vi "main 9th.vi"() -> ()   [LabVIEW 2015]
uses:
  Abort.vi
panel:
  out "number of function calls":i32
  out "External Trigger":bool
  out "x-y":u32
  in  "Live Image Display 2":refnum<k7>(container)
  in  "Live Image Display":refnum<k7>(container)
  in  "Initial guess values 2":dbl[](array[numeric])
  in  "Fitting Results Save Path 2":string[](array[string])
  out "Current File Num":u16
  out "Two Cameras ?":bool
  out "3":u32
  out "2":u32
  out "5":u32
  out "4":u32
  out "From OD fit?":bool
  in  "Fitting Results Save Path":string[](array[string])
  in  "Initial guess values":dbl[](array[numeric])
  out "Latest image data":dbl[][](array[numeric])
  in  "Fitting Type":u16(ring)
  in  "Force Guess?":bool
  in  "Abort":bool
  in  "FFT Auto?":bool[](array[boolean]) caption="Auto?"
  in  "Ring":u16(ring) items=["Atom", "Light", "Dark", "OD"]
  in  "Select Cam Fit":bool[](array[boolean])
  in  "Binning Average?":bool caption="Average?"
  in  "FFT Process":bool caption="Process"
  in  "Threshold":dbl
  out "Label":string[](array[string])
  in  "Pics to show in IJ":bool[][](array[boolean])
  out "Trigger":bool
  in  "Save Fit":bool
  out "best fit parameters 2":dbl[][](array[numeric])
  in  "Binning Enabled":bool
  in  "Binning":u8[](array[numeric])
  out "ROI Width":u16[](array[numeric])
  out "ROI Height":u16[](array[numeric])
  out "best fit parameters":dbl[][](array[numeric])
  in  "Reset Cam Buffer":bool
  out "OD image":u16[][](graph)
  out "XY图":cluster{i32[], dbl[]}[](graph)
  in  "OD fit":bool caption="Open"
  in  "OD Num":i32
  out "Fitting...":bool
  in  "Exit":bool
  out "XY图 2":cluster{i32[], dbl[]}[](graph)
  in  "Fit":bool
  in  "Open File":bool
  in  "Auto Fit":bool
  in  "Stop":bool
  in  "Aquire":bool
  in  "Fitting Config":bool
  in  "Camera Config":bool
  in  "Initialize":bool
  # "Cam1"
  # "Cam2"
  # "Atom"
  # "Light"
  # "Dark"
  # "OD"
  # "FFT and Low Pass"
  # "Na"
  # "Rb"
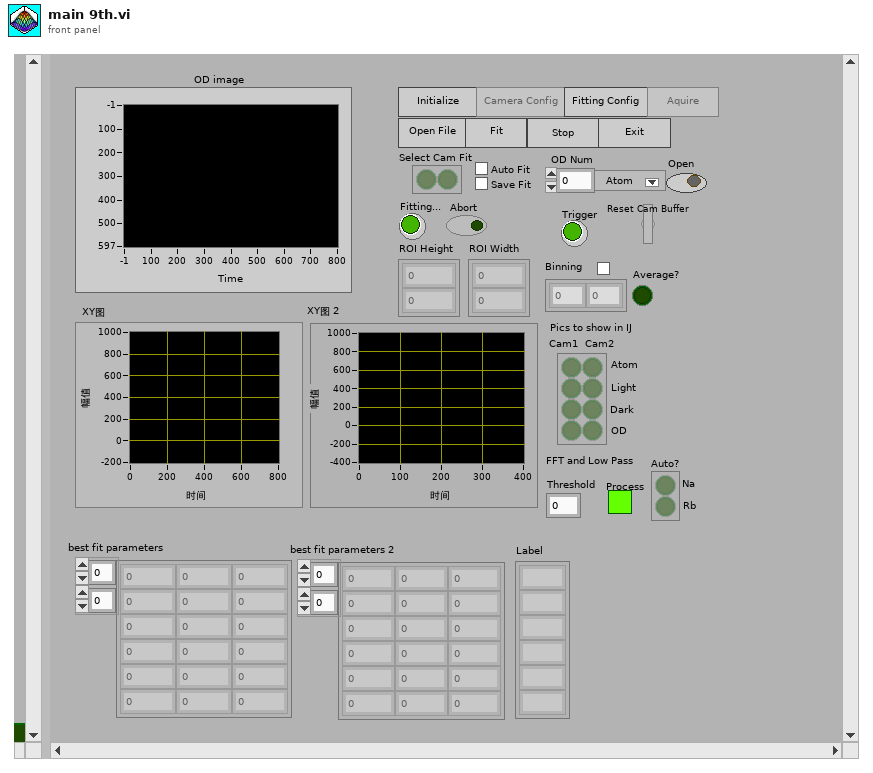
[diagram p1: front panel]
types:
  T1 = enum8{"Enabled", "Disabled", "Disabled and Grayed Out"}
  T2 = enum16{"Left Button", "Center Button", "Right Button", "Window Close"}
  T3 = typedef "Image Type" = u32
  T4 = typedef "IMAQ Image.ctl" = refnum<image>
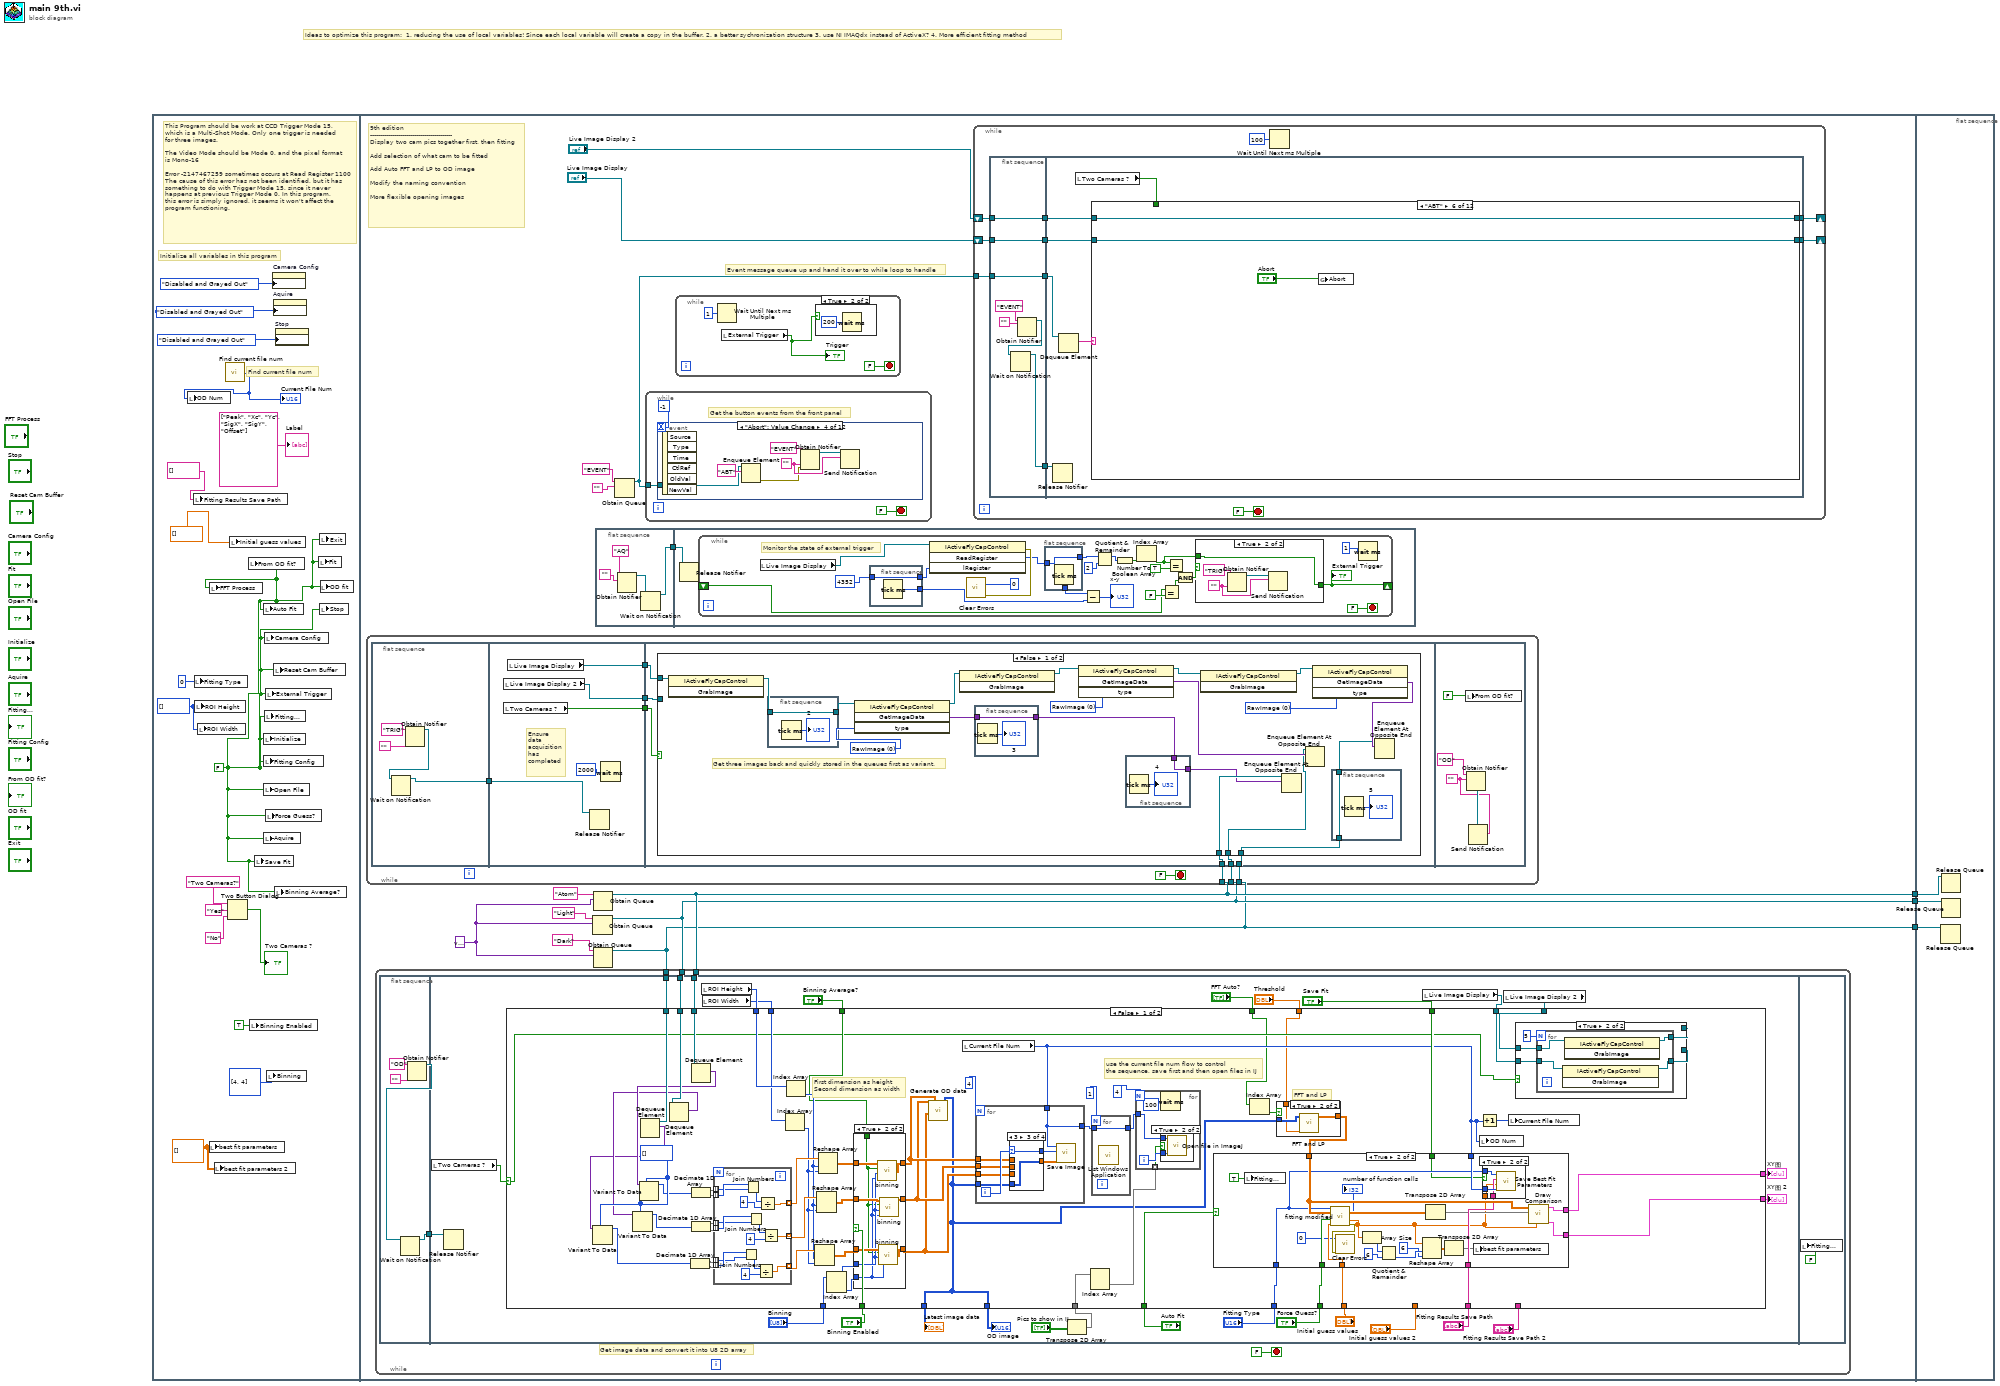
[diagram p0: block diagram]
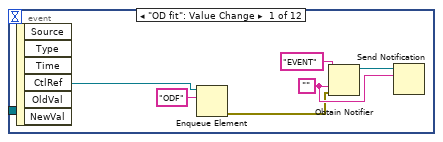
[diagram p3: hidden frame]
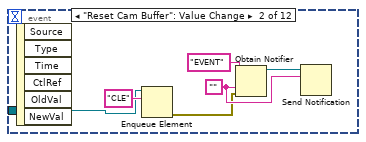
[diagram p4: hidden frame]
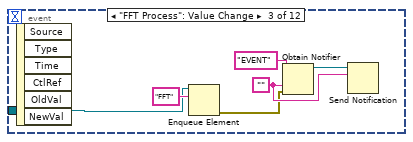
[diagram p5: hidden frame]
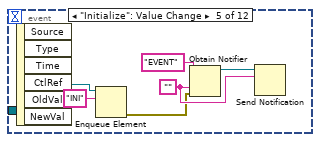
[diagram p6: hidden frame]
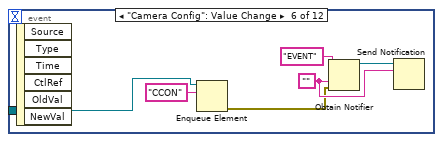
[diagram p7: hidden frame]
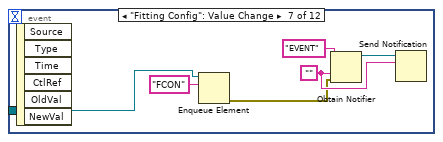
[diagram p8: hidden frame]
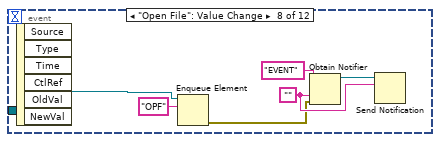
[diagram p9: hidden frame]
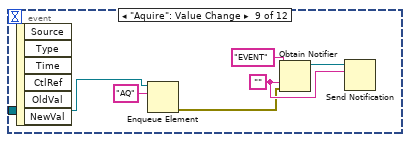
[diagram p10: hidden frame]
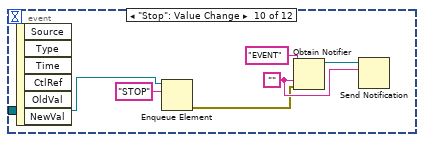
[diagram p11: hidden frame]
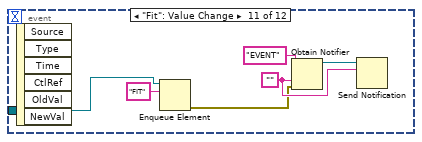
[diagram p12: hidden frame]
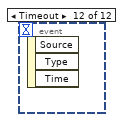
[diagram p13: hidden frame]
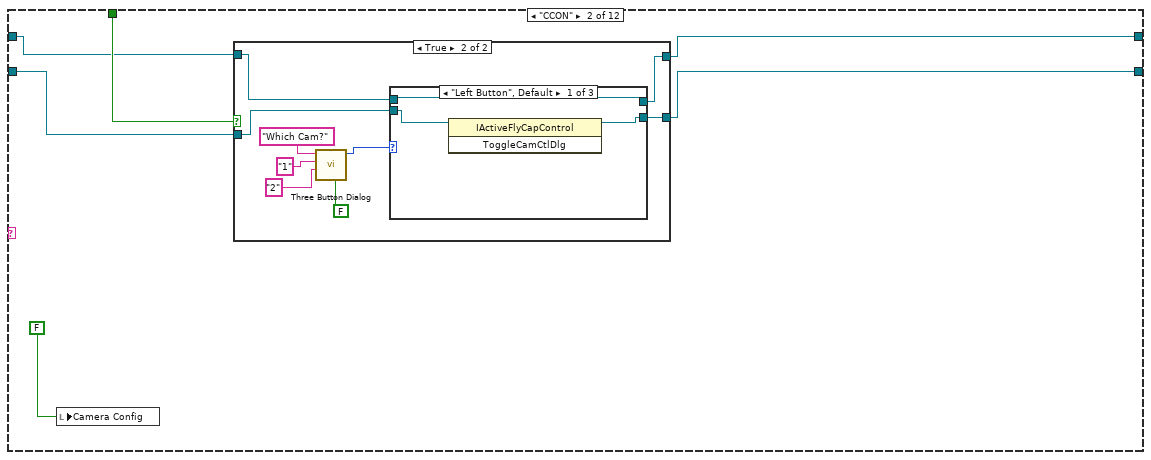
[diagram p15: hidden frame]
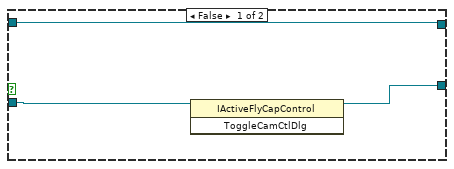
[diagram p16: hidden frame]
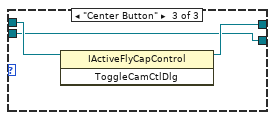
[diagram p18: hidden frame]
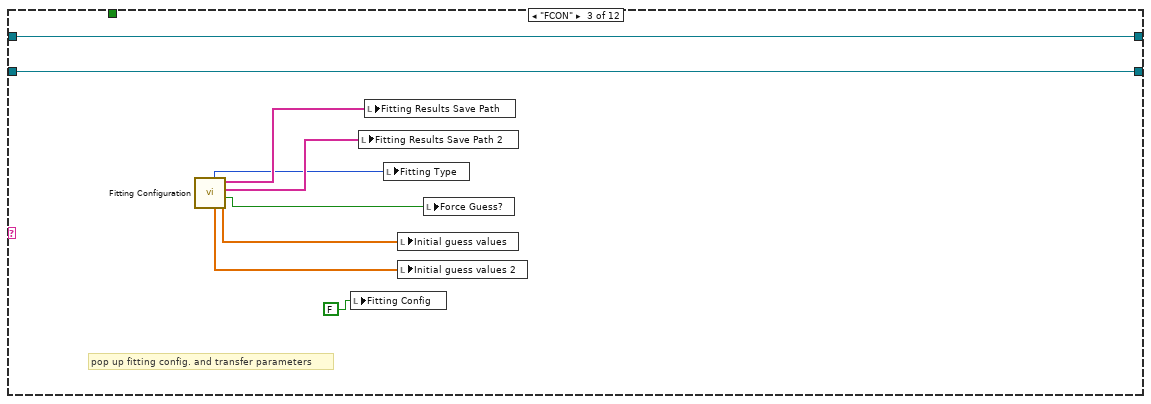
[diagram p19: hidden frame]
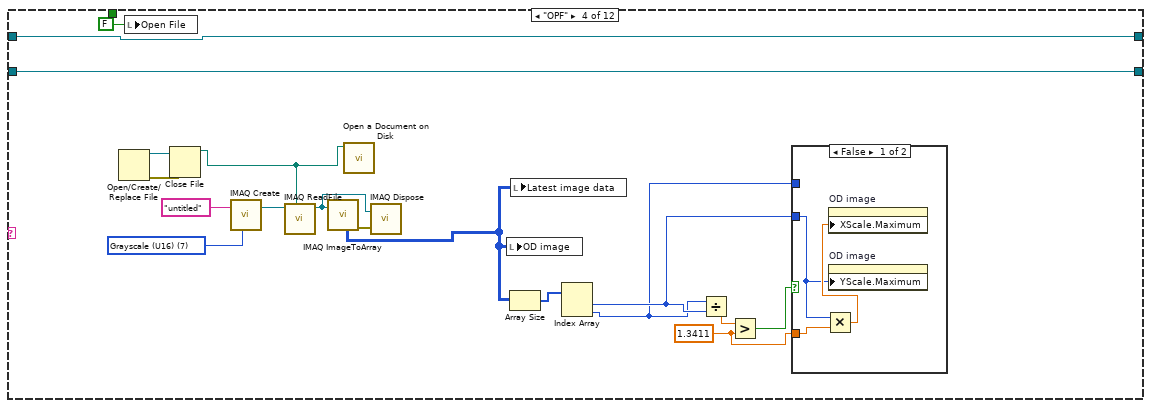
[diagram p20: hidden frame]
diagram:
  # "Ideas to optimize this program:  1. reducing the use of local variables! Since each local variable will create a copy in the buffer. 2. a better sychronization structure 3. use NI IMAQdx instead of ActiveX? 4. More efficient fitting method"
  n1 = flat-sequence {
    tunnel: [w29] -> w3
    tunnel: [w28] -> w2
    tunnel: [w27] -> w1
    tunnel: w3 -> [w1041]
    tunnel: w2 -> [w1040]
    tunnel: w1 -> [w1039]
    frame #0 {
      w6 = dbl[][] [] ("best fit parameters")
      w10 = u16[] [] ("ROI Height")
      w5 = FALSE ("Aquire")
      # "This Program should be work at CCD Trigger Mode 15,\nwhich is a Multi-Shot Mode. Only one trigger is needed\nfor three images. \n\nThe Video Mode should be Mode 0, and the pixel format\nis Mono-16\n\nError -2147467259 sometimes occurs at Read Register 1100\nThe cause of this error has not been identified, but it has\nsomething to do with Trigger Mode 15, since it never \nhappens at previous Trigger Mode 0. In this program,\nthis error is simply ignored, it seems it won't affect the \nprogram functioning."
      # "Find current file num"
      # "Initialize all variables in this program"
      n2 = local write "Fitting Results Save Path"(string[] [] ("Fitting Results Save Path")) -> ()
      n3 = local write "Fitting Type"(0 ("OD num")) -> ()
      n4 = local write "ROI Height"(w10) -> ()
      n5 = local write "ROI Width"(w10) -> ()
      n6 = local write "best fit parameters"(w6) -> ()
      n7 = local write "FFT Process"(w5) -> ()
      n8 = local write "best fit parameters 2"(w6) -> ()
      n9 = call "Find current file num.vi"() -> ("Current File Num"=w4:u16)  [unwired: 2 in]
      "Current File Num" <- w4
      n10 = local write "OD Num"(w4) -> ()
      n11 = Two Button Dialog(message="Two Cameras?" ("消息"), 1:"No" ("F按钮名称（“取消”）"), 2:"Yes" ("T按钮名称（“确定”）")) -> (T button?=→"Two Cameras ?":bool)
      n12 = local write "Initial guess values"(dbl[] [] ("Best fit parameters")) -> ()
      n13 = local write "From OD fit?"(w5) -> ()
      n14 = local write "Binning Enabled"(TRUE ("Binning Enabled")) -> ()
      n15 = local write "Save Fit"(w5) -> ()
      n16 = local write "Auto Fit"(w5) -> ()
      n17 = local write "Initialize"(w5) -> ()
      n18 = local write "Fitting Config"(w5) -> ()
      n19 = local write "Open File"(w5) -> ()
      n20 = local write "Aquire"(w5) -> ()
      n21 = local write "Camera Config"(w5) -> ()
      n22 = local write "Fitting..."(w5) -> ()
      n23 = local write "Force Guess?"(w5) -> ()
      n24 = local write "External Trigger"(w5) -> ()
      n25 = local write "Binning"(u8[] [4, 4] ("Binning")) -> ()
      n26 = property on="Camera Config" class="Bool (strict)"("DisabledEnum"=T1."Disabled and Grayed Out" ("禁用")) -> ()  [unwired: 2 in, 2 out]
      n27 = property on="Aquire" class="Bool (strict)"("DisabledEnum"=T1."Disabled and Grayed Out" ("禁用")) -> ()  [unwired: 2 in, 2 out]
      n28 = local write "Reset Cam Buffer"(w5) -> ()
      n29 = local write "Binning Average?"(w5) -> ()
      n30 = property on="Stop" class="Bool (strict)"("DisabledEnum"=T1."Disabled and Grayed Out" ("禁用")) -> ()  [unwired: 2 in, 2 out]
      n31 = local write "Fit"(w5) -> ()
      n32 = local write "Exit"(w5) -> ()
      n33 = local write "Stop"(w5) -> ()
      n34 = local write "OD fit"(w5) -> ()
      "Label" <- string[] ["Peak", "Xc", "Yc", "SigX", "SigY", "Offset"] ("Label")
    }
    frame #1 {
      w23 = variant
      # "9th edition\n-----------------------------------------\nDisplay two cam pics together first, then fitting\n\nAdd selection of what cam to be fitted\n\nAdd Auto FFT and LP to OD image\n\nModify the naming convention\n\nMore flexible opening images"
      # "Event message queue up and hand it over to while loop to handle"
      n35 = Obtain Queue(name (unnamed)="Light" ("名称（未命名）"), element data type=w23) -> (queue out=w28:refnum<queue>)  [unwired: 3 in, 2 out]
      n36 = Obtain Queue(name (unnamed)="Atom" ("名称（未命名）"), element data type=w23) -> (queue out=w29:refnum<queue>)  [unwired: 3 in, 2 out]
      n37 = Obtain Queue(name (unnamed)="Dark" ("名称（未命名）"), element data type=w23) -> (queue out=w27:refnum<queue>)  [unwired: 3 in, 2 out]
      n38 = while {
        tunnel: w29 -> [w949]
        tunnel: w28 -> [w948]
        tunnel: w27 -> [w947]
        stop <- FALSE stop-if-true
        n39 = flat-sequence {
          tunnel: [w951] -> w950
          tunnel: w950 -> [w959]
          tunnel: [w958] -> w945
          tunnel: [w957] -> w944
          tunnel: [w956] -> w943
          tunnel: w949 -> [w965]
          tunnel: w948 -> [w964]
          tunnel: w947 -> [w963]
          tunnel: w945 -> [w962]
          tunnel: w944 -> [w961]
          tunnel: w943 -> [w960]
          frame #0 {
            n40 = Obtain Notifier(name (unnamed)="TRIG" ("名称（未命名）"), notification data type="") -> (notifier out=w952:refnum<notifier>)  [unwired: 2 in, 2 out]
            n41 = Wait on Notification(notifier=w952) -> (notifier out=w951:refnum<notifier>)  [unwired: 3 in, 3 out]
          }
          frame #1 {
            # "Ensure\ndata\nacquisition\nhas \ncompleted"
            n42 = local read "Live Image Display 2"() -> (w957:refnum<k7>)
            n43 = local read "Two Cameras ?"() -> (w956:bool)
            n44 = local read "Live Image Display"() -> (w958:refnum<k7>)
            n45 = Release Notifier(notifier=w959) -> ()  [unwired: 2 in, 3 out]
            n46 = Wait (ms)(milliseconds to wait=u32 2000) -> ()  [unwired: 1 out]
          }
          frame #2 {
            n47 = case shown="False" w960 {
              tunnel: w965 -> [w983 w998]
              tunnel: w964 -> [w974 w997]
              tunnel: w963 -> [w971 w996]
              tunnel: w962 -> [w967 w994]
              tunnel: w961 -> [_ w993]
              frame False {
                w969 = 0 items=["RawImage", "ColorProcessedImage"] ("type")
                w970 = 0 items=["RawImage", "ColorProcessedImage"] ("type")
                w984 = 0 items=["RawImage", "ColorProcessedImage"] ("type")
                # "Get three images back and quickly stored in the queues first as variant."
                n48 = invoke class="IActiveFlyCapControl" method="GrabImage"(reference=w967) -> (reference out=w966:refnum<k7>)  [unwired: 2 in, 2 out]
                n49 = flat-sequence {
                  tunnel: w966 -> [w987]
                  tunnel: [w987] -> w981
                  frame #0 {
                    n50 = Tick Count (ms)() -> (millisecond timer value=→"2":u32)
                  }
                }
                n51 = invoke class="IActiveFlyCapControl" method="GetImageData"(reference=w981, "type"=w984) -> (reference out=w978:refnum<k7>, "GetImageData"=w980:variant)  [unwired: 2 in, 2 out]
                n52 = invoke class="IActiveFlyCapControl" method="GrabImage"(reference=w978) -> (reference out=w977:refnum<k7>)  [unwired: 2 in, 2 out]
                n53 = flat-sequence {
                  tunnel: [w985] -> w979
                  tunnel: w980 -> [w985]
                  frame #0 {
                    n54 = Tick Count (ms)() -> (millisecond timer value=→"3":u32)
                  }
                }
                n55 = invoke class="IActiveFlyCapControl" method="GetImageData"(reference=w977, "type"=w970) -> (reference out=w976:refnum<k7>, "GetImageData"=w975:variant)  [unwired: 2 in, 2 out]
                n56 = flat-sequence {
                  tunnel: w979 -> [w992]
                  tunnel: [w992] -> w982
                  frame #0 {
                    n57 = Tick Count (ms)() -> (millisecond timer value=→"4":u32)
                  }
                }
                n58 = invoke class="IActiveFlyCapControl" method="GrabImage"(reference=w976) -> (reference out=w973:refnum<k7>)  [unwired: 2 in, 2 out]
                n59 = Enqueue Element At Opposite End(queue=w983, element=w982) -> ()  [unwired: 2 in, 3 out]
                n60 = Enqueue Element At Opposite End(queue=w974, element=w975) -> ()  [unwired: 2 in, 3 out]
                n61 = invoke class="IActiveFlyCapControl" method="GetImageData"(reference=w973, "type"=w969) -> ("GetImageData"=w972:variant)  [unwired: 2 in, 3 out]
                n62 = flat-sequence {
                  tunnel: w971 -> [w989]
                  tunnel: [w989] -> w968
                  frame #0 {
                    n63 = Tick Count (ms)() -> (millisecond timer value=→"5":u32)
                  }
                }
                n64 = Enqueue Element At Opposite End(queue=w968, element=w972) -> ()  [unwired: 2 in, 3 out]
              }
              frame True {
                # "Since element is added at the front of the queue, queue cam2 first then cam1"
                n65 = for {
                  N: 2 -> [_]
                  tunnel: w998 -> [w1004]
                  tunnel: w997 -> [w1003]
                  tunnel: w996 -> [w1002]
                  tunnel: w994 -> [w1000]
                  tunnel: w993 -> [w999]
                  i -> [w1001]
                  n66 = case shown="0, Default" w1001 {
                    tunnel: w1004 -> [w1008 w1024]
                    tunnel: w1003 -> [w1007 w1023]
                    tunnel: w1002 -> [w1006 w1022]
                    tunnel: w1000 -> [_ w1021]
                    tunnel: w999 -> [w1005 _]
                    frame 0, Default {
                      w1011 = 0 items=["RawImage", "ColorProcessedImage"] ("type")
                      w1012 = 0 items=["RawImage", "ColorProcessedImage"] ("type")
                      w1019 = 0 items=["RawImage", "ColorProcessedImage"] ("type")
                      # "Get three images back and quickly stored in the queues first as variant."
                      n67 = invoke class="IActiveFlyCapControl" method="GrabImage"(reference=w1005) -> (reference out=w1010:refnum<k7>)  [unwired: 2 in, 2 out]
                      n68 = invoke class="IActiveFlyCapControl" method="GetImageData"(reference=w1010, "type"=w1019) -> (reference out=w1018:refnum<k7>, "GetImageData"=w1009:variant)  [unwired: 2 in, 2 out]
                      n69 = invoke class="IActiveFlyCapControl" method="GrabImage"(reference=w1018) -> (reference out=w1017:refnum<k7>)  [unwired: 2 in, 2 out]
                      n70 = invoke class="IActiveFlyCapControl" method="GetImageData"(reference=w1017, "type"=w1012) -> (reference out=w1016:refnum<k7>, "GetImageData"=w1015:variant)  [unwired: 2 in, 2 out]
                      n71 = invoke class="IActiveFlyCapControl" method="GrabImage"(reference=w1016) -> (reference out=w1014:refnum<k7>)  [unwired: 2 in, 2 out]
                      n72 = invoke class="IActiveFlyCapControl" method="GetImageData"(reference=w1014, "type"=w1011) -> ("GetImageData"=w1013:variant)  [unwired: 2 in, 3 out]
                      n73 = Enqueue Element At Opposite End(queue=w1008, element=w1009) -> ()  [unwired: 2 in, 3 out]
                      n74 = Enqueue Element At Opposite End(queue=w1007, element=w1015) -> ()  [unwired: 2 in, 3 out]
                      n75 = Enqueue Element At Opposite End(queue=w1006, element=w1013) -> ()  [unwired: 2 in, 3 out]
                    }
                    frame 1 {
                      w1027 = 0 items=["RawImage", "ColorProcessedImage"] ("type")
                      w1028 = 0 items=["RawImage", "ColorProcessedImage"] ("type")
                      w1034 = 0 items=["RawImage", "ColorProcessedImage"] ("type")
                      # "Get three images back and quickly stored in the queues first as variant."
                      n76 = invoke class="IActiveFlyCapControl" method="GrabImage"(reference=w1021) -> (reference out=w1026:refnum<k7>)  [unwired: 2 in, 2 out]
                      n77 = invoke class="IActiveFlyCapControl" method="GetImageData"(reference=w1026, "type"=w1034) -> (reference out=w1033:refnum<k7>, "GetImageData"=w1025:variant)  [unwired: 2 in, 2 out]
                      n78 = invoke class="IActiveFlyCapControl" method="GrabImage"(reference=w1033) -> (reference out=w1032:refnum<k7>)  [unwired: 2 in, 2 out]
                      n79 = invoke class="IActiveFlyCapControl" method="GetImageData"(reference=w1032, "type"=w1028) -> (reference out=w1031:refnum<k7>, "GetImageData"=w1030:variant)  [unwired: 2 in, 2 out]
                      n80 = invoke class="IActiveFlyCapControl" method="GrabImage"(reference=w1031) -> (reference out=w1020:refnum<k7>)  [unwired: 2 in, 2 out]
                      n81 = invoke class="IActiveFlyCapControl" method="GetImageData"(reference=w1020, "type"=w1027) -> ("GetImageData"=w1029:variant)  [unwired: 2 in, 3 out]
                      n82 = Enqueue Element At Opposite End(queue=w1024, element=w1025) -> ()  [unwired: 2 in, 3 out]
                      n83 = Enqueue Element At Opposite End(queue=w1023, element=w1030) -> ()  [unwired: 2 in, 3 out]
                      n84 = Enqueue Element At Opposite End(queue=w1022, element=w1029) -> ()  [unwired: 2 in, 3 out]
                    }
                  }
                }
              }
            }
          }
          frame #3 {
            w1036 = ""
            n85 = local write "From OD fit?"(FALSE ("From OD fit?")) -> ()
            n86 = Obtain Notifier(name (unnamed)="OD" ("名称（未命名）"), notification data type=w1036) -> (notifier out=w1038:refnum<notifier>)  [unwired: 2 in, 2 out]
            n87 = Send Notification(notification=w1036, notifier=w1038) -> ()  [unwired: 1 in, 2 out]
          }
        }
      }
      n88 = while {
        tunnel: w29 -> [w451]
        tunnel: w28 -> [w450]
        tunnel: w27 -> [w449]
        stop <- FALSE stop-if-true
        # "Get image data and convert it into U8 2D array"
        n89 = flat-sequence {
          tunnel: [w453] -> w452
          tunnel: w452 -> [w481]
          tunnel: w451 -> [w484]
          tunnel: w450 -> [w483]
          tunnel: w449 -> [w482]
          frame #0 {
            n90 = Obtain Notifier(name (unnamed)="OD" ("名称（未命名）"), notification data type="") -> (notifier out=w454:refnum<notifier>)  [unwired: 2 in, 2 out]
            n91 = Wait on Notification(notifier=w454) -> (notifier out=w453:refnum<notifier>)  [unwired: 3 in, 3 out]
          }
          frame #1 {
            n92 = local read "Two Cameras ?"() -> (w480:bool)
            n93 = Release Notifier(notifier=w481) -> ()  [unwired: 2 in, 3 out]
            n94 = local read "ROI Height"() -> (w477:u16[])
            n95 = local read "ROI Width"() -> (w476:u16[])
            n96 = Transpose 2D Array(2D array="Pics to show in IJ") -> (transposed array=w463:bool[][])
            n97 = local read "Live Image Display"() -> (w459:refnum<k7>)
            n98 = local read "Live Image Display 2"() -> (w460:refnum<k7>)
            n99 = case shown="False" w480 {
              selector: w480 -> [w490 _]
              tunnel: w484 -> [w542 w682]
              tunnel: w483 -> [w541 w681]
              tunnel: w482 -> [w540 w680]
              tunnel: "Binning" -> [w509 w679]
              tunnel: "Binning Enabled" -> [w508 w678]
              tunnel: w477 -> [w507 w677]
              tunnel: w476 -> [w506 w676]
              tunnel: [w489 w675] -> w475
              tunnel: [w489 w675] -> w474
              tunnel: "Auto Fit" -> [w505 w674]
              tunnel: "Initial guess values" -> [w504 w663]
              tunnel: "Force Guess?" -> [w503 w664]
              tunnel: "Fitting Type" -> [w502 w673]
              tunnel: "Fitting Results Save Path" -> [w501 w660]
              tunnel: [w499 w656] -> w468
              tunnel: [w498 w655] -> w467
              tunnel: "Fitting Results Save Path 2" -> [_ w659]
              tunnel: "Initial guess values 2" -> [_ w658]
              tunnel: "Save Fit" -> [w497 w662]
              tunnel: w463 -> [w496 w671]
              tunnel: "Binning Average?" -> [w494 w670]
              tunnel: w460 -> [w492 w668]
              tunnel: w459 -> [w491 w669]
              tunnel: "Threshold" -> [w485 w647]
              tunnel: "FFT Auto?" -> [w488 w646]
              frame False {
                w525 = u8[] []
                # "FFT and LP"
                # "First dimension as height\nSecond dimension as width"
                # "use the current file num flow to control \nthe sequence, save first and then open files in IJ"
                n100 = Dequeue Element(queue=w540) -> (element=w523:variant)  [unwired: 2 in, 3 out]
                n101 = Variant To Data(type=w525, Variant=w523) -> (data=w520:u8[])  [unwired: 1 in, 1 out]
                n102 = Dequeue Element(queue=w541) -> (element=w524:variant)  [unwired: 2 in, 3 out]
                n103 = Variant To Data(type=w525, Variant=w524) -> (data=w521:u8[])  [unwired: 1 in, 1 out]
                n104 = Decimate 1D Array(w520) -> (w531:u8[], w530:u8[])
                n105 = Dequeue Element(queue=w542) -> (element=w526:variant)  [unwired: 2 in, 3 out]
                n106 = Variant To Data(type=w525, Variant=w526) -> (data=w522:u8[])  [unwired: 1 in, 1 out]
                n107 = Decimate 1D Array(w522) -> (w535:u8[], w534:u8[])
                n108 = Decimate 1D Array(w521) -> (w533:u8[], w532:u8[])
                n109 = for {
                  tunnel: [w589] -> w529 mode=indexing
                  tunnel: w535 -> [w579] mode=indexing
                  tunnel: w534 -> [w580] mode=indexing
                  tunnel: w533 -> [w581] mode=indexing
                  tunnel: w532 -> [w582] mode=indexing
                  tunnel: w531 -> [w583] mode=indexing
                  tunnel: w530 -> [w584] mode=indexing
                  tunnel: [w578] -> w528 mode=indexing
                  tunnel: [w577] -> w527 mode=indexing
                  n110 = Join Numbers(hi=w584, lo=w583) -> ((hi.lo)=w586:u16)
                  n111 = Join Numbers(hi=w580, lo=w579) -> ((hi.lo)=w591:u16)
                  n112 = Join Numbers(hi=w582, lo=w581) -> ((hi.lo)=w588:u16)
                  n113 = Divide(x=w586, y=u16 4) -> (x/y=w577:dbl)
                  n114 = Divide(x=w591, y=u16 4) -> (x/y=w589:dbl)
                  n115 = Divide(x=w588, y=u16 4) -> (x/y=w578:dbl)
                }
                n116 = Index Array(array=w506) -> (element=w518:u16)  [unwired: 1 in]
                n117 = Index Array(array=w507) -> (element=w519:u16)  [unwired: 1 in]
                n118 = Reshape Array(w527, w519, w518) -> (w512:dbl[][])
                n119 = Reshape Array(w528, w519, w518) -> (w514:dbl[][])
                n120 = Reshape Array(w529, w519, w518) -> (w516:dbl[][])
                n121 = Index Array(array=w509) -> (element #1=w511:u8, element #2=w510:u8)  [unwired: 2 in]
                n122 = case shown="True" w508 {
                  tunnel: [w567 w575] -> w517
                  tunnel: w516 -> [w567 w576]
                  tunnel: [w566 w573] -> w515
                  tunnel: w514 -> [w566 w574]
                  tunnel: [w565 w572] -> w513
                  tunnel: w512 -> [w565 w571]
                  tunnel: w511 -> [_ w570]
                  tunnel: w510 -> [_ w569]
                  tunnel: w494 -> [_ w568]
                  frame False {
                  }
                  frame True {
                    n123 = call "binning.vi"("y binning"=w569, "x binning"=w570, "Average?"=w568, "data in"=w576) -> ("data out"=w575:dbl[][])
                    n124 = call "binning.vi"("y binning"=w569, "x binning"=w570, "Average?"=w568, "data in"=w571) -> ("data out"=w572:dbl[][])
                    n125 = call "binning.vi"("y binning"=w569, "x binning"=w570, "Average?"=w568, "data in"=w574) -> ("data out"=w573:dbl[][])
                  }
                }
                n126 = call "Generate OD data.vi"("dark"=w513, "light"=w515, "atom"=w517) -> ("OD image"=w489:u16[][])  [unwired: 3 in]
                n127 = local read "Current File Num"() -> (w493:u16)
                n128 = for {
                  N: 4 -> [_]
                  tunnel: w517 -> [w636]
                  tunnel: w515 -> [w635]
                  tunnel: w513 -> [w634]
                  tunnel: w489 -> [w633]
                  tunnel: w493 -> [w630]
                  tunnel: [w630] -> w536
                  i -> [w637]
                  n129 = case shown="3" w637 {
                    selector: w637 -> [w639 w641 w643 w645]
                    tunnel: w636 -> [w638 _ _ _]
                    tunnel: w635 -> [_ _ _ w644]
                    tunnel: w634 -> [_ w640 _ _]
                    tunnel: w633 -> [_ _ w642 _]
                    tunnel: [w639 w641 w643 w645] -> w632
                    tunnel: [w638 w640 w642 w644] -> w631
                    frame 0, Default {
                    }
                    frame 2 {
                    }
                    frame 3 {
                    }
                    frame 1 {
                    }
                  }
                  n130 = call "Save Image.vi"("Data"=w631, "Process Index"=w632, "Current File Num"=w630) -> ()  [unwired: 9 in]
                }
                n131 = Index Array(array=w496) -> (element=w495:bool[])  [unwired: 2 in]
                n132 = for {
                  N: 1 -> [_]
                  tunnel: w536 -> [w592]
                  tunnel: [w592] -> w538
                  n133 = call "List Windows Application.vi"() -> ()  [unwired: 1 in]
                }
                n134 = for {
                  N: 4 -> [_]
                  tunnel: w538 -> [w596]
                  tunnel: w495 -> [w593] mode=indexing
                  i -> [w595]
                  n135 = case shown="True" w593 {
                    tunnel: w596 -> [_ w598]
                    tunnel: w595 -> [_ w597]
                    frame False {
                    }
                    frame True {
                      n136 = call "Open file in ImageJ.vi"("Process Index"=w597, "Current File Num"=w598) -> ()  [unwired: 10 in]
                    }
                  }
                  n137 = Wait (ms)(milliseconds to wait=u32 100) -> ()  [unwired: 1 out]
                }
                n138 = Index Array(array=w488) -> (element=w487:bool)  [unwired: 1 in]
                n139 = case shown="True" w487 {
                  tunnel: w489 -> [w544 w547]
                  tunnel: [w544 w546] -> w486
                  tunnel: w485 -> [_ w545]
                  frame False {
                  }
                  frame True {
                    n140 = call "FFT and LP.vi"("Threshold"=w545, "Data In"=w547) -> ("Data Out"=w546:dbl[][])  [unwired: 9 in]
                  }
                }
                n141 = case shown="True" w505 {
                  tunnel: w486 -> [w603 w624]
                  tunnel: w493 -> [_ w612]
                  tunnel: [w602 w623] -> w499
                  tunnel: [w601 w622] -> w498
                  tunnel: w504 -> [_ w621]
                  tunnel: w503 -> [_ w620]
                  tunnel: w502 -> [_ w610]
                  tunnel: w501 -> [_ w611]
                  tunnel: w497 -> [_ w609]
                  frame False {
                    n142 = Transpose 2D Array(2D array=w603) -> (transposed array=w600:dbl[][])
                    n143 = call "Draw Comparison.vi"("Best Fit Parameters"=dbl[] [0.0, 0.0, 0.0, 0.0, 0.0], "Best Fit"=w600, "Raw Data"=w603) -> ("Vertical Comparison"=w601:cluster{i32[], dbl[]}[], "Horizontal Comparison"=w602:cluster{i32[], dbl[]}[])  [unwired: 6 in]
                  }
                  frame True {
                    n144 = local write "Fitting..."(TRUE ("Fitting...")) -> ()
                    n145 = call "fitting modified.vi"("fitting type"=w610, "2D data"=w624, "force guess?"=w620, "intial guess value"=w621) -> ("number of function calls"=→"number of function calls":i32, "best fit"=w625:dbl[][], "best fit parameters"=w604:dbl[], "error out"=w614:errorcluster)  [unwired: 8 in]
                    n146 = call <vilib>:"Clear Errors.vi"("error in (no error)"=w614, "specific error code to clear (0: all)"=0) -> ()  [unwired: 4 in, 2 out]
                    n147 = Array Size(array=w604) -> (size(s)=w618:i32)
                    n148 = Quotient & Remainder(x=w618, y=6) -> (floor(x/y)=w607:i32)  [unwired: 1 out]
                    n149 = Reshape Array(w604, w607, 6 ("dimension size")) -> (w619:dbl[][])
                    n150 = Transpose 2D Array(2D array=w625) -> (transposed array=w605:dbl[][])
                    n151 = Transpose 2D Array(2D array=w619) -> (transposed array=w608:dbl[][])
                    n152 = local write "best fit parameters"(w608) -> ()
                    n153 = case shown="True" w609 {
                      tunnel: w612 -> [_ w629]
                      tunnel: w611 -> [_ w628]
                      tunnel: w604 -> [_ w627]
                      tunnel: w610 -> [_ w626]
                      frame False {
                      }
                      frame True {
                        n154 = call "Save Best Fit Parameters.vi"("Current File Num"=w629, "Best Fit Parameters"=w627, "Fitting Results Save Path"=w628, "Fitting Type"=w626) -> ()  [unwired: 8 in]
                      }
                    }
                    n155 = call "Draw Comparison.vi"("Best Fit Parameters"=w604, "Best Fit"=w605, "Raw Data"=w624) -> ("Vertical Comparison"=w622:cluster{i32[], dbl[]}[], "Horizontal Comparison"=w623:cluster{i32[], dbl[]}[])  [unwired: 6 in]
                  }
                }
                n156 = local write "OD Num"(w493) -> ()
                n157 = Increment(x=w493) -> (x+1=w500:u16)
                n158 = local write "Current File Num"(w500) -> ()
                n159 = case shown="True" w490 {
                  tunnel: w491 -> [w552 w560]
                  tunnel: [w548 w558] -> _
                  tunnel: w492 -> [w550 w557]
                  tunnel: [w551 w556] -> _
                  frame False {
                    n160 = for {
                      N: 5 -> [_]
                      tunnel: [w555] -> w548
                      tunnel: w552 -> [w554]
                      tunnel: [w553] -> w551
                      tunnel: w550 -> [w553]
                      n161 = invoke class="IActiveFlyCapControl" method="GrabImage"(reference=w554) -> (reference out=w555:refnum<k7>)  [unwired: 2 in, 2 out]
                    }
                  }
                  frame True {
                    n162 = for {
                      N: 5 -> [_]
                      tunnel: w560 -> [w564]
                      tunnel: [w563] -> w558
                      tunnel: w557 -> [w562]
                      tunnel: [w561] -> w556
                      n163 = invoke class="IActiveFlyCapControl" method="GrabImage"(reference=w564) -> (reference out=w563:refnum<k7>)  [unwired: 2 in, 2 out]
                      n164 = invoke class="IActiveFlyCapControl" method="GrabImage"(reference=w562) -> (reference out=w561:refnum<k7>)  [unwired: 2 in, 2 out]
                    }
                  }
                }
              }
              frame True {
                # "FFT and LP"
                n165 = for {
                  N: 2 -> [_]
                  tunnel: w682 -> [w852]
                  tunnel: w681 -> [w851]
                  tunnel: w680 -> [w850]
                  tunnel: w679 -> [w849]
                  tunnel: w678 -> [w848]
                  tunnel: w677 -> [w847]
                  tunnel: w676 -> [w846]
                  tunnel: [w811] -> w675
                  tunnel: w674 -> [w809]
                  tunnel: w673 -> [w808]
                  tunnel: w662 -> [_]
                  tunnel: w671 -> [w845] mode=indexing
                  tunnel: w670 -> [w844]
                  shift-right: [w811] -> w650
                  shift-left: _ -> [w810]
                  tunnel: [w810] -> w651
                  tunnel: [w809] -> w665
                  tunnel: [w808] -> w661
                  tunnel: [w807] -> w653
                  i -> [w806]
                  w829 = u8[] []
                  # "First dimension as height\nSecond dimension as width"
                  # "use the current file num flow to control \nthe sequence, save first and then open files in IJ"
                  n166 = Dequeue Element(queue=w850) -> (element=w827:variant)  [unwired: 2 in, 3 out]
                  n167 = Variant To Data(type=w829, Variant=w827) -> (data=w824:u8[])  [unwired: 1 in, 1 out]
                  n168 = Decimate 1D Array(w824) -> (w835:u8[], w834:u8[])
                  n169 = Dequeue Element(queue=w851) -> (element=w828:variant)  [unwired: 2 in, 3 out]
                  n170 = Variant To Data(type=w829, Variant=w828) -> (data=w825:u8[])  [unwired: 1 in, 1 out]
                  n171 = Decimate 1D Array(w825) -> (w837:u8[], w836:u8[])
                  n172 = Dequeue Element(queue=w852) -> (element=w830:variant)  [unwired: 2 in, 3 out]
                  n173 = Variant To Data(type=w829, Variant=w830) -> (data=w826:u8[])  [unwired: 1 in, 1 out]
                  n174 = Decimate 1D Array(w826) -> (w839:u8[], w838:u8[])
                  n175 = for {
                    tunnel: [w877] -> w833 mode=indexing
                    tunnel: w839 -> [w867] mode=indexing
                    tunnel: w838 -> [w868] mode=indexing
                    tunnel: w837 -> [w869] mode=indexing
                    tunnel: w836 -> [w870] mode=indexing
                    tunnel: w835 -> [w871] mode=indexing
                    tunnel: w834 -> [w872] mode=indexing
                    tunnel: [w866] -> w832 mode=indexing
                    tunnel: [w865] -> w831 mode=indexing
                    n176 = Join Numbers(hi=w872, lo=w871) -> ((hi.lo)=w874:u16)
                    n177 = Join Numbers(hi=w868, lo=w867) -> ((hi.lo)=w879:u16)
                    n178 = Join Numbers(hi=w870, lo=w869) -> ((hi.lo)=w876:u16)
                    n179 = Divide(x=w874, y=u16 4) -> (x/y=w865:dbl)
                    n180 = Divide(x=w879, y=u16 4) -> (x/y=w877:dbl)
                    n181 = Divide(x=w876, y=u16 4) -> (x/y=w866:dbl)
                  }
                  n182 = Index Array(array=w846) -> (element=w822:u16)  [unwired: 1 in]
                  n183 = Index Array(array=w847) -> (element=w823:u16)  [unwired: 1 in]
                  n184 = Index Array(array=w849) -> (element #1=w815:u8, element #2=w814:u8)  [unwired: 2 in]
                  n185 = Reshape Array(w831, w823, w822) -> (w816:dbl[][])
                  n186 = Reshape Array(w832, w823, w822) -> (w818:dbl[][])
                  n187 = Reshape Array(w833, w823, w822) -> (w820:dbl[][])
                  n188 = case shown="True" w848 {
                    tunnel: [w855 w863] -> w821
                    tunnel: w820 -> [w855 w864]
                    tunnel: [w854 w861] -> w819
                    tunnel: w818 -> [w854 w862]
                    tunnel: [w853 w860] -> w817
                    tunnel: w816 -> [w853 w859]
                    tunnel: w815 -> [_ w858]
                    tunnel: w814 -> [_ w857]
                    tunnel: w844 -> [_ w856]
                    frame False {
                    }
                    frame True {
                      n189 = call "binning.vi"("y binning"=w857, "x binning"=w858, "Average?"=w856, "data in"=w864) -> ("data out"=w863:dbl[][])
                      n190 = call "binning.vi"("y binning"=w857, "x binning"=w858, "Average?"=w856, "data in"=w859) -> ("data out"=w860:dbl[][])
                      n191 = call "binning.vi"("y binning"=w857, "x binning"=w858, "Average?"=w856, "data in"=w862) -> ("data out"=w861:dbl[][])
                    }
                  }
                  n192 = call "Generate OD data.vi"("dark"=w817, "light"=w819, "atom"=w821) -> ("OD image"=w811:u16[][])  [unwired: 3 in]
                  n193 = local read "Current File Num"() -> (w807:u16)
                  n194 = for {
                    N: 4 -> [_]
                    tunnel: w821 -> [w895]
                    tunnel: w819 -> [w894]
                    tunnel: w817 -> [w893]
                    tunnel: w811 -> [w892]
                    tunnel: w807 -> [w889]
                    tunnel: [w889] -> w840
                    tunnel: w806 -> [w887]
                    i -> [w896]
                    n195 = case shown="1" w896 {
                      selector: w896 -> [w898 w900 w902 w904]
                      tunnel: w895 -> [w897 _ _ _]
                      tunnel: w894 -> [_ _ _ w903]
                      tunnel: w893 -> [_ w899 _ _]
                      tunnel: w892 -> [_ _ w901 _]
                      tunnel: [w898 w900 w902 w904] -> w891
                      tunnel: [w897 w899 w901 w903] -> w890
                      frame 0, Default {
                      }
                      frame 2 {
                      }
                      frame 3 {
                      }
                      frame 1 {
                      }
                    }
                    n196 = Increment(x=w891) -> (x+1=w888:i32)
                    n197 = call "Save Image.vi"("Data"=w890, "Na/Rb (0/1)"=w887, "Process Index"=w888, "Current File Num"=w889) -> ()  [unwired: 8 in]
                  }
                  n198 = Negate(x=w806) -> (-x=w813:i32)
                  n199 = Increment(x=w813) -> (x+1=w812:i32)
                  n200 = for {
                    N: w812 -> [_]
                    tunnel: w840 -> [w880]
                    tunnel: [w880] -> w841
                    n201 = call "List Windows Application.vi"() -> ()  [unwired: 1 in]
                  }
                  n202 = for {
                    N: 4 -> [_]
                    tunnel: w841 -> [w884]
                    tunnel: w845 -> [w881] mode=indexing
                    i -> [w883]
                    n203 = Wait (ms)(milliseconds to wait=u32 100) -> ()  [unwired: 1 out]
                    n204 = case shown="True" w881 {
                      tunnel: w884 -> [_ w886]
                      tunnel: w883 -> [_ w885]
                      frame False {
                      }
                      frame True {
                        n205 = call "Open file in ImageJ.vi"("Process Index"=w885, "Current File Num"=w886) -> ()  [unwired: 10 in]
                      }
                    }
                  }
                }
                n206 = Increment(x=w653) -> (x+1=w654:u16)
                n207 = Index Array(array=w646) -> (element #1=w652:bool)  [unwired: 2 in, 1 out]
                n208 = case shown="False" w652 {
                  tunnel: w647 -> [_ w690]
                  tunnel: w651 -> [w687 w689]
                  tunnel: [w687 w688] -> w648
                  frame False {
                  }
                  frame True {
                    n209 = call "FFT and LP.vi"("Threshold"=w690, "Data In"=w689) -> ("Data Out"=w688:dbl[][])  [unwired: 9 in]
                  }
                }
                n210 = case shown="True" w652 {
                  tunnel: w647 -> [_ w686]
                  tunnel: w650 -> [w683 w685]
                  tunnel: [w683 w684] -> w649
                  frame False {
                  }
                  frame True {
                    n211 = call "FFT and LP.vi"("Threshold"=w686, "Data In"=w685) -> ("Data Out"=w684:dbl[][])  [unwired: 9 in]
                  }
                }
                n212 = local write "OD Num"(w653) -> ()
                n213 = local write "Current File Num"(w654) -> ()
                n214 = for {
                  N: 2 -> [_]
                  tunnel: "Select Cam Fit" -> [w710] mode=indexing
                  tunnel: w665 -> [w709]
                  tunnel: w648 -> [w707]
                  tunnel: w649 -> [w706]
                  tunnel: w664 -> [w705]
                  tunnel: w663 -> [w704]
                  tunnel: w662 -> [w703]
                  tunnel: w661 -> [w702]
                  tunnel: w660 -> [w701]
                  tunnel: w659 -> [w700]
                  tunnel: w658 -> [w699]
                  tunnel: w653 -> [w698]
                  tunnel: [w695] -> w656
                  tunnel: [w692] -> w655
                  i -> [w711]
                  w691 = cluster{i32[], dbl[]}[] []
                  n215 = And(x=w710, y=w709) -> (x .and. y?=w708:bool)
                  n216 = case shown="1" w711 {
                    tunnel: w708 -> [w714 w760]
                    tunnel: w707 -> [w717 w759]
                    tunnel: w706 -> [_ w758]
                    tunnel: w705 -> [w721 w753]
                    tunnel: w704 -> [w720 _]
                    tunnel: w703 -> [w719 w755]
                    tunnel: w702 -> [w718 w756]
                    tunnel: w701 -> [w716 _]
                    tunnel: w700 -> [_ w757]
                    tunnel: w699 -> [_ w754]
                    tunnel: w698 -> [w715 w752]
                    tunnel: [w712 w751] -> w694
                    tunnel: [w713 w750] -> w696
                    frame 0, Default {
                      n217 = case shown="False" w714 {
                        tunnel: [w726 w744] -> w713
                        tunnel: [w725 w743] -> w712
                        tunnel: w720 -> [_ w742]
                        tunnel: w721 -> [_ w741]
                        tunnel: w716 -> [_ w740]
                        tunnel: w719 -> [_ w735]
                        tunnel: w718 -> [_ w728]
                        tunnel: w717 -> [w722 w729]
                        tunnel: w715 -> [_ w727]
                        frame False {
                          n218 = Transpose 2D Array(2D array=w722) -> (transposed array=w724:dbl[][])
                          n219 = call "Draw Comparison.vi"("Best Fit Parameters"=dbl[] [0.0, 0.0, 0.0, 0.0, 0.0], "Best Fit"=w724, "Raw Data"=w722) -> ("Vertical Comparison"=w725:cluster{i32[], dbl[]}[], "Horizontal Comparison"=w726:cluster{i32[], dbl[]}[])  [unwired: 6 in]
                        }
                        frame True {
                          n220 = call "fitting modified.vi"("fitting type"=w728, "2D data"=w729, "force guess?"=w741, "intial guess value"=w742) -> ("best fit"=w745:dbl[][], "best fit parameters"=w731:dbl[])  [unwired: 8 in, 2 out]
                          n221 = Array Size(array=w731) -> (size(s)=w738:i32)
                          n222 = Quotient & Remainder(x=w738, y=6) -> (floor(x/y)=w732:i32)  [unwired: 1 out]
                          n223 = Reshape Array(w731, w732, 6 ("dimension size")) -> (w739:dbl[][])
                          n224 = Transpose 2D Array(2D array=w739) -> (transposed array=w734:dbl[][])
                          n225 = local write "best fit parameters"(w734) -> ()
                          n226 = Transpose 2D Array(2D array=w745) -> (transposed array=w730:dbl[][])
                          n227 = local write "Fitting..."(TRUE ("Fitting...")) -> ()
                          n228 = case shown="True" w735 {
                            tunnel: w727 -> [_ w749]
                            tunnel: w728 -> [_ w748]
                            tunnel: w740 -> [_ w746]
                            tunnel: w731 -> [_ w747]
                            frame False {
                            }
                            frame True {
                              n229 = call "Save Best Fit Parameters.vi"("Current File Num"=w749, "Best Fit Parameters"=w747, "Fitting Results Save Path"=w746, "Fitting Type"=w748) -> ()  [unwired: 8 in]
                            }
                          }
                          n230 = call "Draw Comparison.vi"("Best Fit Parameters"=w731, "Best Fit"=w730, "Raw Data"=w729) -> ("Vertical Comparison"=w743:cluster{i32[], dbl[]}[], "Horizontal Comparison"=w744:cluster{i32[], dbl[]}[])  [unwired: 6 in]
                        }
                      }
                    }
                    frame 1 {
                      n231 = case shown="False" w760 {
                        tunnel: w756 -> [_ w767]
                        tunnel: w753 -> [_ w783]
                        tunnel: [w765 w782] -> w750
                        tunnel: [w764 w781] -> w751
                        tunnel: w757 -> [_ w780]
                        tunnel: w754 -> [_ w779]
                        tunnel: w755 -> [_ w774]
                        tunnel: w759 -> [w761 _]
                        tunnel: w758 -> [_ w768]
                        tunnel: w752 -> [_ w766]
                        frame False {
                          n232 = Transpose 2D Array(2D array=w761) -> (transposed array=w763:dbl[][])
                          n233 = call "Draw Comparison.vi"("Best Fit Parameters"=dbl[] [0.0, 0.0, 0.0, 0.0, 0.0], "Best Fit"=w763, "Raw Data"=w761) -> ("Vertical Comparison"=w764:cluster{i32[], dbl[]}[], "Horizontal Comparison"=w765:cluster{i32[], dbl[]}[])  [unwired: 6 in]
                        }
                        frame True {
                          n234 = call "fitting modified.vi"("fitting type"=w767, "2D data"=w768, "force guess?"=w783, "intial guess value"=w779) -> ("best fit"=w784:dbl[][], "best fit parameters"=w770:dbl[])  [unwired: 8 in, 2 out]
                          n235 = Array Size(array=w770) -> (size(s)=w777:i32)
                          n236 = Quotient & Remainder(x=w777, y=6) -> (floor(x/y)=w771:i32)  [unwired: 1 out]
                          n237 = case shown="True" w774 {
                            tunnel: w766 -> [_ w788]
                            tunnel: w767 -> [_ w787]
                            tunnel: w780 -> [_ w786]
                            tunnel: w770 -> [_ w785]
                            frame False {
                            }
                            frame True {
                              n238 = call "Save Best Fit Parameters.vi"("Current File Num"=w788, "Best Fit Parameters"=w785, "Fitting Results Save Path"=w786, "Fitting Type"=w787) -> ()  [unwired: 8 in]
                            }
                          }
                          n239 = Reshape Array(w770, w771, 6 ("dimension size")) -> (w778:dbl[][])
                          n240 = Transpose 2D Array(2D array=w778) -> (transposed array=→"best fit parameters 2":dbl[][])
                          n241 = Transpose 2D Array(2D array=w784) -> (transposed array=w769:dbl[][])
                          n242 = local write "Fitting..."(TRUE ("Fitting...")) -> ()
                          n243 = call "Draw Comparison.vi"("Best Fit Parameters"=w770, "Best Fit"=w769, "Raw Data"=w768) -> ("Vertical Comparison"=w781:cluster{i32[], dbl[]}[], "Horizontal Comparison"=w782:cluster{i32[], dbl[]}[])  [unwired: 6 in]
                        }
                      }
                    }
                  }
                  n244 = feedback #1(w691) -> (w697:cluster{i32[], dbl[]}[])
                  n245 = Insert Into Array(array=w697, new element=w696) -> (w695:cluster{i32[], dbl[]}[])  [unwired: 1 in]
                  n246 = feedback-in #1(w695) -> ()
                  n247 = feedback #2(w691) -> (w693:cluster{i32[], dbl[]}[])
                  n248 = Insert Into Array(array=w693, new element=w694) -> (w692:cluster{i32[], dbl[]}[])  [unwired: 1 in]
                  n249 = feedback-in #2(w692) -> ()
                }
                n250 = local read "Two Cameras ?"() -> (w657:bool)
                n251 = case shown="True" w657 {
                  tunnel: w668 -> [w793 w801]
                  tunnel: [w789 w799] -> _
                  tunnel: w669 -> [w791 w798]
                  tunnel: [w792 w797] -> _
                  frame False {
                    n252 = for {
                      N: 5 -> [_]
                      tunnel: [w796] -> w789
                      tunnel: w793 -> [w795]
                      tunnel: [w794] -> w792
                      tunnel: w791 -> [w794]
                      n253 = invoke class="IActiveFlyCapControl" method="GrabImage"(reference=w795) -> (reference out=w796:refnum<k7>)  [unwired: 2 in, 2 out]
                    }
                  }
                  frame True {
                    n254 = for {
                      N: 5 -> [_]
                      tunnel: w801 -> [w805]
                      tunnel: [w804] -> w799
                      tunnel: w798 -> [w803]
                      tunnel: [w802] -> w797
                      n255 = invoke class="IActiveFlyCapControl" method="GrabImage"(reference=w805) -> (reference out=w804:refnum<k7>)  [unwired: 2 in, 2 out]
                      n256 = invoke class="IActiveFlyCapControl" method="GrabImage"(reference=w803) -> (reference out=w802:refnum<k7>)  [unwired: 2 in, 2 out]
                    }
                  }
                }
              }
            }
            "Latest image data" <- w475
            "OD image" <- w474
            "XY图" <- w468
            "XY图 2" <- w467
          }
          frame #2 {
            n257 = local write "Fitting..."(FALSE ("Fitting...")) -> ()
          }
        }
      }
      n258 = flat-sequence {
        tunnel: [w906] -> w33
        tunnel: w33 -> [w910]
        frame #0 {
          n259 = Obtain Notifier(name (unnamed)="AQ" ("名称（未命名）"), notification data type="") -> (notifier out=w908:refnum<notifier>)  [unwired: 2 in, 2 out]
          n260 = Wait on Notification(notifier=w908) -> (notifier out=w906:refnum<notifier>)  [unwired: 3 in, 3 out]
        }
        frame #1 {
          n261 = Release Notifier(notifier=w910) -> ()  [unwired: 2 in, 3 out]
          n262 = while {
            shift-right: [w922] -> _
            shift-left: _ -> [w921]
            stop <- FALSE stop-if-true
            # "Monitor the state of external trigger"
            n263 = local read "Live Image Display"() -> (w933:refnum<k7>)
            n264 = flat-sequence {
              tunnel: [w937] -> w915
              tunnel: u32 4352 ("lRegister") -> [w937]
              tunnel: [w936] -> w912
              frame #0 {
                n265 = Tick Count (ms)() -> (millisecond timer value=w936:u32)
              }
            }
            n266 = invoke class="IActiveFlyCapControl" method="ReadRegister"(reference=w933, "lRegister"=w915) -> (error out=w919:errorcluster, "ReadRegister"=w917:u32)  [unwired: 2 in, 2 out]
            n267 = call <vilib>:"Clear Errors.vi"("error in (no error)"=w919, "specific error code to clear (0: all)"=0) -> ()  [unwired: 4 in, 2 out]
            n268 = flat-sequence {
              tunnel: w917 -> [w935]
              tunnel: [w935] -> w916
              tunnel: [w934] -> w913
              frame #0 {
                n269 = Tick Count (ms)() -> (millisecond timer value=w934:u32)
              }
            }
            n270 = Subtract(x=w913, y=w912) -> (x-y=→"x-y":u32)
            n271 = Quotient & Remainder(x=w916, y=u32 2) -> (x-y*floor(x/y)=w931:u32)  [unwired: 1 out]
            n272 = Number To Boolean Array(number=w931) -> (Boolean array=w930:bool[])
            n273 = Index Array(array=w930) -> (element=w924:bool)  [unwired: 1 in]
            n274 = Equal?(x=w921, y=FALSE) -> (x = y?=w927:bool)
            n275 = Equal?(x=w924, y=TRUE) -> (x = y?=w926:bool)
            n276 = And(x=w926, y=w927) -> (x .and. y?=w925:bool)
            n277 = case shown="True" w925 {
              tunnel: w924 -> [w938 w939]
              tunnel: [w938 w939] -> w922
              frame False {
              }
              frame True {
                w940 = ""
                n278 = Obtain Notifier(name (unnamed)="TRIG" ("名称（未命名）"), notification data type=w940) -> (notifier out=w941:refnum<notifier>)  [unwired: 2 in, 2 out]
                n279 = Send Notification(notification=w940, notifier=w941) -> ()  [unwired: 1 in, 2 out]
              }
            }
            "External Trigger" <- w922
            n280 = Wait (ms)(milliseconds to wait=u32 1) -> ()  [unwired: 1 out]
          }
        }
      }
      n281 = Obtain Queue(name (unnamed)="EVENT" ("名称（未命名）"), element data type="") -> (queue out=w24:refnum<queue>)  [unwired: 3 in, 2 out]
      n282 = while {
        tunnel: w24 -> [w38]
        stop <- FALSE stop-if-true
        # "Get the button events from the front panel"
        n283 = event shown="[3] \"Abort\": Value Change" {
          selector: _ -> [_ _ _ _ _ _ _ _ _ _ _ _]
          dyn-events: _ -> [_ _ _ _ _ _ _ _ _ _ _ _]
          timeout: -1 -> [_ _ _ _ _ _ _ _ _ _ _ _]
          tunnel: w38 -> [w41 w47 w53 w59 w66 w71 w77 w83 w89 w95 w101 _]
          event "OD fit": Value Change {
            w44 = ""
            n284 = event-data() -> ()  [unwired: 1 in, 6 out]
            n285 = Enqueue Element(queue=w41, element="ODF") -> (error out=w42:errorcluster)  [unwired: 2 in, 2 out]
            n286 = Obtain Notifier(name (unnamed)="EVENT" ("名称（未命名）"), notification data type=w44, error in (no error)=w42) -> (notifier out=w45:refnum<notifier>)  [unwired: 1 in, 2 out]
            n287 = Send Notification(notification=w44, notifier=w45) -> ()  [unwired: 1 in, 2 out]
          }
          event "Reset Cam Buffer": Value Change {
            w50 = ""
            n288 = event-data() -> ()  [unwired: 1 in, 6 out]
            n289 = Enqueue Element(queue=w47, element="CLE") -> (error out=w48:errorcluster)  [unwired: 2 in, 2 out]
            n290 = Obtain Notifier(name (unnamed)="EVENT" ("名称（未命名）"), notification data type=w50, error in (no error)=w48) -> (notifier out=w51:refnum<notifier>)  [unwired: 1 in, 2 out]
            n291 = Send Notification(notification=w50, notifier=w51) -> ()  [unwired: 1 in, 2 out]
          }
          event "FFT Process": Value Change {
            w56 = ""
            n292 = event-data() -> ()  [unwired: 1 in, 6 out]
            n293 = Enqueue Element(queue=w53, element="FFT") -> (error out=w54:errorcluster)  [unwired: 2 in, 2 out]
            n294 = Obtain Notifier(name (unnamed)="EVENT" ("名称（未命名）"), notification data type=w56, error in (no error)=w54) -> (notifier out=w57:refnum<notifier>)  [unwired: 1 in, 2 out]
            n295 = Send Notification(notification=w56, notifier=w57) -> ()  [unwired: 1 in, 2 out]
          }
          event "Abort": Value Change {
            w62 = ""
            n296 = event-data() -> ()  [unwired: 1 in, 6 out]
            n297 = Enqueue Element(queue=w59, element="ABT") -> (error out=w60:errorcluster)  [unwired: 2 in, 2 out]
            n298 = Obtain Notifier(name (unnamed)="EVENT" ("名称（未命名）"), notification data type=w62, error in (no error)=w60) -> (notifier out=w63:refnum<notifier>)  [unwired: 1 in, 2 out]
            n299 = Send Notification(notification=w62, notifier=w63) -> ()  [unwired: 1 in, 2 out]
          }
          event "Initialize": Value Change {
            w68 = ""
            n300 = event-data() -> ()  [unwired: 1 in, 6 out]
            n301 = Enqueue Element(queue=w66, element="INI") -> (error out=w65:errorcluster)  [unwired: 2 in, 2 out]
            n302 = Obtain Notifier(name (unnamed)="EVENT" ("名称（未命名）"), notification data type=w68, error in (no error)=w65) -> (notifier out=w69:refnum<notifier>)  [unwired: 1 in, 2 out]
            n303 = Send Notification(notification=w68, notifier=w69) -> ()  [unwired: 1 in, 2 out]
          }
          event "Camera Config": Value Change {
            w74 = ""
            n304 = event-data() -> ()  [unwired: 1 in, 6 out]
            n305 = Enqueue Element(queue=w71, element="CCON") -> (error out=w72:errorcluster)  [unwired: 2 in, 2 out]
            n306 = Obtain Notifier(name (unnamed)="EVENT" ("名称（未命名）"), notification data type=w74, error in (no error)=w72) -> (notifier out=w75:refnum<notifier>)  [unwired: 1 in, 2 out]
            n307 = Send Notification(notification=w74, notifier=w75) -> ()  [unwired: 1 in, 2 out]
          }
          event "Fitting Config": Value Change {
            w80 = ""
            n308 = event-data() -> ()  [unwired: 1 in, 6 out]
            n309 = Enqueue Element(queue=w77, element="FCON") -> (error out=w78:errorcluster)  [unwired: 2 in, 2 out]
            n310 = Obtain Notifier(name (unnamed)="EVENT" ("名称（未命名）"), notification data type=w80, error in (no error)=w78) -> (notifier out=w81:refnum<notifier>)  [unwired: 1 in, 2 out]
            n311 = Send Notification(notification=w80, notifier=w81) -> ()  [unwired: 1 in, 2 out]
          }
          event "Open File": Value Change {
            w86 = ""
            n312 = event-data() -> ()  [unwired: 1 in, 6 out]
            n313 = Enqueue Element(queue=w83, element="OPF") -> (error out=w84:errorcluster)  [unwired: 2 in, 2 out]
            n314 = Obtain Notifier(name (unnamed)="EVENT" ("名称（未命名）"), notification data type=w86, error in (no error)=w84) -> (notifier out=w87:refnum<notifier>)  [unwired: 1 in, 2 out]
            n315 = Send Notification(notification=w86, notifier=w87) -> ()  [unwired: 1 in, 2 out]
          }
          event "Aquire": Value Change {
            w92 = ""
            n316 = event-data() -> ()  [unwired: 1 in, 6 out]
            n317 = Enqueue Element(queue=w89, element="AQ") -> (error out=w90:errorcluster)  [unwired: 2 in, 2 out]
            n318 = Obtain Notifier(name (unnamed)="EVENT" ("名称（未命名）"), notification data type=w92, error in (no error)=w90) -> (notifier out=w93:refnum<notifier>)  [unwired: 1 in, 2 out]
            n319 = Send Notification(notification=w92, notifier=w93) -> ()  [unwired: 1 in, 2 out]
          }
          event "Stop": Value Change {
            w98 = ""
            n320 = event-data() -> ()  [unwired: 1 in, 6 out]
            n321 = Enqueue Element(queue=w95, element="STOP") -> (error out=w96:errorcluster)  [unwired: 2 in, 2 out]
            n322 = Obtain Notifier(name (unnamed)="EVENT" ("名称（未命名）"), notification data type=w98, error in (no error)=w96) -> (notifier out=w99:refnum<notifier>)  [unwired: 1 in, 2 out]
            n323 = Send Notification(notification=w98, notifier=w99) -> ()  [unwired: 1 in, 2 out]
          }
          event "Fit": Value Change {
            w104 = ""
            n324 = event-data() -> ()  [unwired: 1 in, 6 out]
            n325 = Enqueue Element(queue=w101, element="FIT") -> (error out=w102:errorcluster)  [unwired: 2 in, 2 out]
            n326 = Obtain Notifier(name (unnamed)="EVENT" ("名称（未命名）"), notification data type=w104, error in (no error)=w102) -> (notifier out=w105:refnum<notifier>)  [unwired: 1 in, 2 out]
            n327 = Send Notification(notification=w104, notifier=w105) -> ()  [unwired: 1 in, 2 out]
          }
          event Timeout {
            n328 = event-data() -> ()  [unwired: 1 in, 3 out]
          }
        }
      }
      n329 = while {
        stop <- FALSE stop-if-true
        n330 = Wait Until Next ms Multiple(millisecond multiple=u32 1) -> ()  [unwired: 1 out]
        n331 = local read "External Trigger"() -> (w34:bool)
        "Trigger" <- w34
        n332 = case shown="True" w34 {
          frame False {
          }
          frame True {
            n333 = Wait (ms)(milliseconds to wait=u32 200) -> ()  [unwired: 1 out]
          }
        }
      }
      n334 = while {
        tunnel: w24 -> [w115]
        shift-right: [w111] -> _
        shift-left: "Live Image Display" -> [w112]
        shift-right: [w110] -> _
        shift-left: "Live Image Display 2" -> [w108]
        stop <- FALSE stop-if-true
        n335 = flat-sequence {
          tunnel: [w121] -> w117
          tunnel: w115 -> [w120]
          tunnel: [w120] -> w114
          tunnel: [w119] -> w113
          tunnel: w112 -> [w119]
          tunnel: [w118] -> w109
          tunnel: w108 -> [w118]
          tunnel: w117 -> [w132]
          tunnel: w114 -> [w131]
          tunnel: w113 -> [w129]
          tunnel: [w128] -> w111
          tunnel: [w127] -> w110
          tunnel: w109 -> [w126]
          frame #0 {
            n336 = Obtain Notifier(name (unnamed)="EVENT" ("名称（未命名）"), notification data type="") -> (notifier out=w122:refnum<notifier>)  [unwired: 2 in, 2 out]
            n337 = Wait on Notification(notifier=w122) -> (notifier out=w121:refnum<notifier>)  [unwired: 3 in, 3 out]
          }
          frame #1 {
            n338 = Release Notifier(notifier=w132) -> ()  [unwired: 2 in, 3 out]
            n339 = Dequeue Element(queue=w131) -> (element=w130:string)  [unwired: 2 in, 3 out]
            n340 = local read "Two Cameras ?"() -> (w125:bool)
            n341 = case shown="\"ABT\"" w130 {
              tunnel: w129 -> [w134 w139 w168 w178 w196 w200 w223 w287 w297 w342 w398 w430]
              tunnel: [w134 w138 w168 w178 w196 w200 w222 w286 w297 w342 w392 w429] -> w128
              tunnel: [w133 w136 w167 w177 w197 w201 w219 w285 w296 w341 w393 w425] -> w127
              tunnel: w126 -> [w133 w135 w167 w177 w197 w201 w218 w284 w296 w341 w394 w426]
              tunnel: w125 -> [_ w137 _ _ _ _ w220 w283 _ _ w395 w427]
              frame Default {
              }
              frame "CCON" {
                n342 = local write "Camera Config"(FALSE ("Camera Config")) -> ()
                n343 = case shown="True" w137 {
                  tunnel: w139 -> [w143 w150]
                  tunnel: [w142 w149] -> w138
                  tunnel: [w141 w147] -> w136
                  tunnel: w135 -> [w141 w148]
                  frame False {
                    n344 = invoke class="IActiveFlyCapControl" method="ToggleCamCtlDlg"(reference=w143) -> (reference out=w142:refnum<k7>)  [unwired: 2 in, 2 out]
                  }
                  frame True {
                    n345 = call <vilib>:"Three Button Dialog.vi"("Allow user to close window? (TRUE)"=FALSE, "Center Button Text (\"No\")"="2" ("F按钮名称（“取消”）"), "Left Button Text (\"Yes\")"="1" ("T按钮名称（“确定”）"), "message"="Which Cam?" ("消息")) -> ("Which Button?"=w151:T2)  [unwired: 7 in]
                    n346 = case shown="\"Left Button\", Default" w151 {
                      tunnel: w150 -> [w155 w157 w158]
                      tunnel: [w154 w157 w158] -> w149
                      tunnel: w148 -> [w153 w156 w159]
                      tunnel: [w153 w156 w160] -> w147
                      frame "Left Button", Default {
                        n347 = invoke class="IActiveFlyCapControl" method="ToggleCamCtlDlg"(reference=w155) -> (reference out=w154:refnum<k7>)  [unwired: 2 in, 2 out]
                      }
                      frame "Right Button" {
                      }
                      frame "Center Button" {
                        n348 = invoke class="IActiveFlyCapControl" method="ToggleCamCtlDlg"(reference=w159) -> (reference out=w160:refnum<k7>)  [unwired: 2 in, 2 out]
                      }
                    }
                  }
                }
              }
              frame "FCON" {
                # "pop up fitting config. and transfer parameters"
                n349 = call "Fitting Configuration.vi"() -> ("Na intial guess"=w162:dbl[], "Force Guess？"=w163:bool, "Na Fitting Results Save Path"=w165:string[], "Rb Fitting Results Save Path"=w166:string[], "Rb intial guess"=w161:dbl[], "Fitting Type"=w164:u16)  [unwired: 6 in]
                n350 = local write "Fitting Config"(FALSE ("Fitting Config")) -> ()
                n351 = local write "Fitting Results Save Path 2"(w165) -> ()
                n352 = local write "Fitting Results Save Path"(w166) -> ()
                n353 = local write "Fitting Type"(w164) -> ()
                n354 = local write "Initial guess values"(w162) -> ()
                n355 = local write "Initial guess values 2"(w161) -> ()
                n356 = local write "Force Guess?"(w163) -> ()
              }
              frame "OPF" {
                w173 = 1.3411 ("y")
                w180 = T3 7 items=["Grayscale (U8)", "Grayscale (I16)", "Grayscale (SGL)", "Complex (CSG)", "RGB (U32)", "HSL (U32)", "RGB (U64)", "Grayscale (U16)"] ("Image Type")
                n357 = Open/Create/Replace File() -> (refnum out=w186:refnum<file>, error out=w185:errorcluster)  [unwired: 6 in, 1 out]
                n358 = local write "Open File"(FALSE ("Open File")) -> ()
                n359 = Close File(refnum=w186, error in=w185) -> (path=w187:path)  [unwired: 1 out]
                n360 = call "IMAQ Create"("Image Name"="untitled", "Image Type"=w180) -> ("New Image"=w181:T4)  [unwired: 3 in, 1 out]
                n361 = call "IMAQ ReadFile"("File Path"=w187, "Image"=w181) -> ("Image Out"=w182:T4)  [unwired: 5 in, 4 out]
                n362 = call "IMAQ ImageToArray"("Image"=w182) -> ("Image Pixels (U16)"=w170:u16[][], "error out"=w183:errorcluster)  [unwired: 3 in, 3 out]
                n363 = call <vilib>:"Open a Document on Disk.vi"("document path"=w187) -> ()  [unwired: 6 in, 1 out]
                n364 = call "IMAQ Dispose"("Image"=w182, "error in (no error)"=w183) -> ()  [unwired: 4 in, 1 out]
                n365 = local write "OD image"(w170) -> ()
                n366 = Array Size(array=w170) -> (size(s)=w176:i32[])
                n367 = local write "Latest image data"(w170) -> ()
                n368 = Index Array(array=w176) -> (element #1=w172:i32, element #2=w171:i32)  [unwired: 2 in]
                n369 = Divide(x=w171, y=w172) -> (x/y=w175:dbl)
                n370 = Greater?(x=w175, y=w173) -> (0:w174:bool)
                n371 = case shown="False" w174 {
                  tunnel: w172 -> [w188 _]
                  tunnel: w173 -> [w190 w193]
                  tunnel: w171 -> [_ w191]
                  frame False {
                    n372 = Multiply(x=w188, y=w190) -> (x*y=w189:dbl)
                    n373 = property on="OD image" class="IntGraph (strict)"("XScale.Maximum"=w189) -> ()  [unwired: 2 in, 2 out]
                    n374 = property on="OD image" class="IntGraph (strict)"("YScale.Maximum"=w188) -> ()  [unwired: 2 in, 2 out]
                  }
                  frame True {
                    n375 = Divide(x=w191, y=w193) -> (x/y=w192:dbl)
                    n376 = property on="OD image" class="IntGraph (strict)"("XScale.Maximum"=w191) -> ()  [unwired: 2 in, 2 out]
                    n377 = property on="OD image" class="IntGraph (strict)"("YScale.Maximum"=w192) -> ()  [unwired: 2 in, 2 out]
                  }
                }
              }
              frame "FFT" {
                n378 = local read "Latest image data"() -> (w199:dbl[][])
                n379 = local read "Threshold"() -> (w194:dbl)
                n380 = call "FFT and LP.vi"("Threshold"=w194, "Data In"=w199) -> ("Data Out"=w198:dbl[][])  [unwired: 9 in]
                n381 = local write "Latest image data"(w198) -> ()
                n382 = local write "OD image"(w198) -> ()
                n383 = local write "FFT Process"(FALSE ("FFT Process")) -> ()
              }
              frame "ABT" {
                n384 = global write "Abort.vi" "Abort"("Abort") -> ()
              }
              frame "AQ" {
                w213 = 1.3411 ("y")
                w228 = ""
                n385 = Obtain Notifier(name (unnamed)="AQ" ("名称（未命名）"), notification data type=w228) -> (notifier out=w227:refnum<notifier>)  [unwired: 2 in, 2 out]
                n386 = case shown="True" w220 {
                  tunnel: w223 -> [w246 w274]
                  tunnel: [w245 w273] -> w222
                  tunnel: [w244 w263] -> w219
                  tunnel: w218 -> [w244 w264]
                  tunnel: [w239 w256] -> w205
                  tunnel: [w240 w257] -> w208
                  frame False {
                    w241 = 0
                    # "Width"
                    # "Height"
                    # "Get Current ROI size"
                    # "Start the camera"
                    n387 = property class="IActiveFlyCapControl"(reference=w246, "Start"=1) -> (reference out=w245:refnum<k7>)  [unwired: 1 in, 1 out]
                    n388 = invoke class="IActiveFlyCapControl" method="ReadRegister"(reference=w246, "lRegister"=u32 8204) -> ("ReadRegister"=w248:u32)  [unwired: 2 in, 3 out]
                    n389 = Number To Hexadecimal String(2:w248) -> (0:w252:string)  [unwired: 1 in]
                    n390 = String Length(string=w252) -> (length=w249:i32)
                    n391 = Subtract(x=w249, y=4) -> (x-y=w251:i32)
                    n392 = String Subset(string=w252, offset (0)=w251) -> (substring=w253:string)  [unwired: 1 in]
                    n393 = String Subset(string=w252, length (rest)=w251) -> (substring=w254:string)  [unwired: 1 in]
                    n394 = Hexadecimal String To Number(string=w253) -> (number=w242:u32)  [unwired: 2 in, 1 out]
                    n395 = Hexadecimal String To Number(string=w254) -> (number=w243:u32)  [unwired: 2 in, 1 out]
                    n396 = Build Array(w242, w241) -> (w240:u32[])
                    n397 = Build Array(w243, w241) -> (w239:u32[])
                  }
                  frame True {
                    w265 = 1 ("Start")
                    # "Width"
                    # "Get Current ROI size"
                    # "Width"
                    # "Height"
                    # "Get Current ROI size"
                    # "Start the camera"
                    n398 = invoke class="IActiveFlyCapControl" method="ReadRegister"(reference=w274, "lRegister"=u32 8204) -> ("ReadRegister"=w276:u32)  [unwired: 2 in, 3 out]
                    n399 = invoke class="IActiveFlyCapControl" method="ReadRegister"(reference=w264, "lRegister"=u32 8204) -> ("ReadRegister"=w268:u32)  [unwired: 2 in, 3 out]
                    n400 = property class="IActiveFlyCapControl"(reference=w264, "Start"=w265) -> (reference out=w263:refnum<k7>)  [unwired: 1 in, 1 out]
                    n401 = property class="IActiveFlyCapControl"(reference=w274, "Start"=w265) -> (reference out=w273:refnum<k7>)  [unwired: 1 in, 1 out]
                    n402 = Number To Hexadecimal String(2:w276) -> (0:w280:string)  [unwired: 1 in]
                    n403 = Number To Hexadecimal String(2:w268) -> (0:w266:string)  [unwired: 1 in]
                    n404 = String Length(string=w280) -> (length=w277:i32)
                    n405 = String Length(string=w266) -> (length=w269:i32)
                    n406 = Subtract(x=w277, y=4) -> (x-y=w279:i32)
                    n407 = Subtract(x=w269, y=4) -> (x-y=w271:i32)
                    n408 = String Subset(string=w280, offset (0)=w279) -> (substring=w281:string)  [unwired: 1 in]
                    n409 = String Subset(string=w280, length (rest)=w279) -> (substring=w282:string)  [unwired: 1 in]
                    n410 = String Subset(string=w266, offset (0)=w271) -> (substring=w262:string)  [unwired: 1 in]
                    n411 = String Subset(string=w266, length (rest)=w271) -> (substring=w272:string)  [unwired: 1 in]
                    n412 = Hexadecimal String To Number(string=w281) -> (number=w261:u32)  [unwired: 2 in, 1 out]
                    n413 = Hexadecimal String To Number(string=w282) -> (number=w259:u32)  [unwired: 2 in, 1 out]
                    n414 = Hexadecimal String To Number(string=w262) -> (number=w260:u32)  [unwired: 2 in, 1 out]
                    n415 = Hexadecimal String To Number(string=w272) -> (number=w258:u32)  [unwired: 2 in, 1 out]
                    n416 = Build Array(w261, w260) -> (w257:u32[])
                    n417 = Build Array(w259, w258) -> (w256:u32[])
                  }
                }
                "ROI Height" <- w208
                "ROI Width" <- w205
                n418 = Send Notification(notification=w228, notifier=w227) -> ()  [unwired: 1 in, 2 out]
                n419 = property on="Stop" class="Bool (strict)"("DisabledEnum"=T1."Enabled" ("禁用")) -> ()  [unwired: 2 in, 2 out]
                n420 = property on="Aquire" class="Bool (strict)"("DisabledEnum"=T1."Disabled and Grayed Out" ("禁用")) -> ()  [unwired: 2 in, 2 out]
                n421 = local write "Aquire"(FALSE ("Initialize")) -> ()
                n422 = property on="Camera Config" class="Bool (strict)"("DisabledEnum"=T1."Disabled and Grayed Out" ("禁用")) -> ()  [unwired: 2 in, 2 out]
                n423 = local read "Binning Enabled"() -> (w210:bool)
                n424 = local read "Binning"() -> (w209:u8[])
                n425 = case shown="False" w210 {
                  tunnel: w209 -> [_ w232]
                  tunnel: [w229 w231] -> w206
                  tunnel: [w229 w230] -> w207
                  frame False {
                    w229 = u8 1 ("Numeric")
                  }
                  frame True {
                    n426 = Index Array(array=w232) -> (element #1=w230:u8, element #2=w231:u8)  [unwired: 2 in]
                  }
                }
                n427 = Divide(x=w205, y=w206) -> (x/y=w203:dbl[])
                n428 = Divide(x=w208, y=w207) -> (x/y=w204:dbl[])
                n429 = Divide(x=w203, y=w204) -> (x/y=w216:dbl[])
                n430 = Array Max & Min(array=w203) -> (max value=w211:dbl)  [unwired: 3 out]
                n431 = Array Max & Min(array=w204) -> (max value=w212:dbl)  [unwired: 3 out]
                n432 = Array Max & Min(array=w216) -> (max index (indices)=w215:i32)  [unwired: 3 out]
                n433 = Greater?(x=w215, y=w213) -> (0:w214:bool)
                n434 = case shown="True" w214 {
                  tunnel: w211 -> [_ _]
                  tunnel: w213 -> [w235 w238]
                  tunnel: w212 -> [w233 w236]
                  frame False {
                    n435 = Multiply(x=w233, y=w235) -> (x*y=w234:dbl)
                    n436 = property on="OD image" class="IntGraph (strict)"("XScale.Maximum"=w234) -> ()  [unwired: 2 in, 2 out]
                    n437 = property on="OD image" class="IntGraph (strict)"("YScale.Maximum"=w233) -> ()  [unwired: 2 in, 2 out]
                  }
                  frame True {
                    n438 = Divide(x=w236, y=w238) -> (x/y=w237:dbl)
                    n439 = property on="OD image" class="IntGraph (strict)"("YScale.Maximum"=w237) -> ()  [unwired: 2 in, 2 out]
                    n440 = property on="OD image" class="IntGraph (strict)"("XScale.Maximum"=w236) -> ()  [unwired: 2 in, 2 out]
                  }
                }
              }
              frame "STOP" {
                w291 = T1."Enabled" ("禁用")
                # "stop the camera"
                n441 = local write "Stop"(FALSE ("Initialize")) -> ()
                n442 = property on="Aquire" class="Bool (strict)"("DisabledEnum"=w291) -> ()  [unwired: 2 in, 2 out]
                n443 = property on="Camera Config" class="Bool (strict)"("DisabledEnum"=w291) -> ()  [unwired: 2 in, 2 out]
                n444 = case shown="False" w283 {
                  tunnel: [w292 w295] -> w285
                  tunnel: w284 -> [w292 w293]
                  frame False {
                  }
                  frame True {
                    n445 = property class="IActiveFlyCapControl"(reference=w293, "Start"=0) -> (reference out=w295:refnum<k7>)  [unwired: 1 in, 1 out]
                  }
                }
                n446 = property class="IActiveFlyCapControl"(reference=w287, "Start"=0) -> (reference out=w286:refnum<k7>)  [unwired: 1 in, 1 out]
                n447 = property on="Stop" class="Bool (strict)"("DisabledEnum"=T1."Disabled and Grayed Out" ("禁用")) -> ()  [unwired: 2 in, 2 out]
              }
              frame "FIT" {
                n448 = stacked-sequence {
                  seq-local: [w299 _ _] -> [_ _ w328]
                  seq-local: [w300 _ _] -> [_ _ w326]
                  seq-local: [w298 _ _] -> [_ w313 w323]
                  frame #0 {
                    n449 = flat-sequence {
                      tunnel: [w304] -> w300
                      tunnel: [w303] -> w299
                      tunnel: [w302] -> w298
                      frame #0 {
                        # "Fit the latest data"
                        n450 = local read "Latest image data"() -> (w304:dbl[][])
                        n451 = local read "Initial guess values"() -> (w306:dbl[])
                        n452 = local read "Force Guess?"() -> (w307:bool)
                        n453 = local read "Fitting Type"() -> (w305:u16)
                        n454 = call "fitting modified.vi"("fitting type"=w305, "2D data"=w304, "force guess?"=w307, "intial guess value"=w306) -> ("best fit"=w303:dbl[][], "best fit parameters"=w302:dbl[])  [unwired: 8 in, 2 out]
                        n455 = local write "Fitting..."(TRUE ("Fit Done")) -> ()
                      }
                      frame #1 {
                        n456 = local write "Fit"(FALSE ("Fit")) -> ()
                        n457 = local write "Fitting..."(FALSE ("Fitting...")) -> ()
                      }
                    }
                  }
                  frame #1 {
                    # "Save best fit parameters"
                    n458 = local read "Fitting Results Save Path"() -> (w319:string[])
                    n459 = local read "Fitting Type"() -> (w320:u16)
                    n460 = local read "From OD fit?"() -> (w318:bool)
                    n461 = Array Size(array=w313) -> (size(s)=w315:i32)
                    n462 = case shown="False" w318 {
                      tunnel: [w321 w322] -> w317
                      frame False {
                        n463 = local read "Current File Num"() -> (w321:u16)
                      }
                      frame True {
                        n464 = local read "OD Num"() -> (w322:i32)
                      }
                    }
                    n465 = Quotient & Remainder(x=w315, y=6) -> (floor(x/y)=w311:i32)  [unwired: 1 out]
                    n466 = Reshape Array(w313, w311, 6 ("dimension size")) -> (w316:dbl[][])
                    n467 = call "Save Best Fit Parameters.vi"("Current File Num"=w317, "Best Fit Parameters"=w313, "Fitting Results Save Path"=w319, "Fitting Type"=w320) -> ()  [unwired: 8 in]
                    n468 = Transpose 2D Array(2D array=w316) -> (transposed array=→"best fit parameters":dbl[][])
                  }
                  frame #2 {
                    # "Draw Comparison"
                    n469 = Transpose 2D Array(2D array=w328) -> (transposed array=w324:dbl[][])
                    n470 = call "Draw Comparison.vi"("Best Fit Parameters"=w323, "Best Fit"=w324, "Raw Data"=w326) -> ("Vertical Comparison"=w330:cluster{i32[], dbl[]}[], "Horizontal Comparison"=w331:cluster{i32[], dbl[]}[])  [unwired: 6 in]
                    n471 = local write "Fit"(FALSE ("Initialize")) -> ()
                    n472 = local write "From OD fit?"(FALSE ("From OD fit?")) -> ()
                    n473 = local write "XY图 2"(w330) -> ()
                    n474 = local write "XY图"(w331) -> ()
                    n475 = local write "Fitting..."(FALSE ("Fit Done")) -> ()
                  }
                }
              }
              frame "ODF" {
                w336 = 1.3411 ("y")
                w362 = T3 7 items=["Grayscale (U8)", "Grayscale (I16)", "Grayscale (SGL)", "Complex (CSG)", "RGB (U32)", "HSL (U32)", "RGB (U64)", "Grayscale (U16)"] ("Image Type")
                w354 = "\\" ("字符串")
                n476 = call "find time.vi"() -> ("day"=w352:string, "month"=w349:string, "year"=w346:string)  [unwired: 3 in]
                n477 = Concatenate Strings("D:\\data\\", w346) -> (w347:string)
                n478 = Less?(x="OD Num", y=100.0) -> (x < y?=w359:bool)
                n479 = Concatenate Strings(w347, w354) -> (w348:string)
                n480 = case shown="False" w359 {
                  tunnel: "OD Num" -> [w379 w381]
                  tunnel: [w378 w380] -> w360
                  frame False {
                    n481 = Number To Decimal String(number=w379) -> (decimal integer string=w378:string)  [unwired: 1 in]
                  }
                  frame True {
                    n482 = Less?(x=w381, y=10.0) -> (x < y?=w382:bool)
                    n483 = case shown="False" w382 {
                      tunnel: w381 -> [w386 w391]
                      tunnel: [w384 w388] -> w380
                      frame False {
                        n484 = Number To Decimal String(number=w386) -> (decimal integer string=w385:string)  [unwired: 1 in]
                        n485 = Concatenate Strings("0" ("字符串"), w385) -> (w384:string)
                      }
                      frame True {
                        n486 = Number To Decimal String(number=w391) -> (decimal integer string=w389:string)  [unwired: 1 in]
                        n487 = Concatenate Strings("00" ("字符串"), w389) -> (w388:string)
                      }
                    }
                  }
                }
                n488 = Concatenate Strings(w348, w349) -> (w350:string)
                n489 = Concatenate Strings(w350, w354) -> (w351:string)
                n490 = Concatenate Strings(w351, w352) -> (w353:string)
                n491 = Concatenate Strings(w353, w354) -> (w355:string)
                n492 = case shown="3" "Ring" {
                  tunnel: ["-0.tif" ("字符串") "-1.tif" ("字符串") "-2.tif" ("字符串") "-OD.tif" ("字符串")] -> w357
                  frame 0, Default {
                  }
                  frame 1 {
                  }
                  frame 2 {
                  }
                  frame 3 {
                  }
                }
                n493 = Concatenate Strings(w355, w360) -> (w356:string)
                n494 = Concatenate Strings(w356, w357) -> (w333:string)
                n495 = String To Path(string=w333) -> (path=w365:path)
                n496 = local write "From OD fit?"(TRUE ("From OD fit?")) -> ()
                n497 = local write "OD fit"(FALSE ("OD fit")) -> ()
                n498 = call "IMAQ Create"("Image Name"="untitled", "Image Type"=w362) -> ("New Image"=w366:T4)  [unwired: 3 in, 1 out]
                n499 = call <vilib>:"Open a Document on Disk.vi"("document path"=w365) -> ()  [unwired: 6 in, 1 out]
                n500 = call "IMAQ ReadFile"("File Path"=w365, "Image"=w366) -> ("Image Out"=w367:T4)  [unwired: 5 in, 4 out]
                n501 = call "IMAQ ImageToArray"("Image"=w367) -> ("Image Pixels (U16)"=w340:u16[][], "error out"=w363:errorcluster)  [unwired: 3 in, 3 out]
                n502 = local write "Latest image data"(w340) -> ()
                n503 = Array Size(array=w340) -> (size(s)=w339:i32[])
                n504 = local write "OD image"(w340) -> ()
                n505 = Index Array(array=w339) -> (element #1=w335:i32, element #2=w334:i32)  [unwired: 2 in]
                n506 = Divide(x=w334, y=w335) -> (x/y=w338:dbl)
                n507 = call "IMAQ Dispose"("Image"=w367, "error in (no error)"=w363) -> ()  [unwired: 4 in, 1 out]
                n508 = Greater?(x=w338, y=w336) -> (0:w337:bool)
                n509 = case shown="False" w337 {
                  tunnel: w334 -> [_ w377]
                  tunnel: w336 -> [w374 w376]
                  tunnel: w335 -> [w372 _]
                  frame False {
                    n510 = Multiply(x=w372, y=w374) -> (x*y=w373:dbl)
                    n511 = property on="OD image" class="IntGraph (strict)"("XScale.Maximum"=w373) -> ()  [unwired: 2 in, 2 out]
                    n512 = property on="OD image" class="IntGraph (strict)"("YScale.Maximum"=w372) -> ()  [unwired: 2 in, 2 out]
                  }
                  frame True {
                    n513 = Divide(x=w377, y=w376) -> (x/y=w375:dbl)
                    n514 = property on="OD image" class="IntGraph (strict)"("XScale.Maximum"=w377) -> ()  [unwired: 2 in, 2 out]
                    n515 = property on="OD image" class="IntGraph (strict)"("YScale.Maximum"=w375) -> ()  [unwired: 2 in, 2 out]
                  }
                }
              }
              frame "INI" {
                n516 = Boolean To (0,1)(Boolean=w395) -> (0, 1=w397:i16)
                n517 = Increment(x=w397) -> (x+1=w396:i16)
                n518 = property on="Camera Config" class="Bool (strict)"("DisabledEnum"=T1."Enabled" ("禁用")) -> ()  [unwired: 2 in, 2 out]
                n519 = for {
                  N: w396 -> [_]
                  tunnel: w398 -> [w406]
                  tunnel: w394 -> [w404]
                  tunnel: [w403] -> w393
                  tunnel: [w402] -> w392
                  i -> [w405]
                  n520 = case shown="1" w405 {
                    selector: w405 -> [w410 w418]
                    tunnel: [w407 w419] -> w403
                    tunnel: w406 -> [w409 w416]
                    tunnel: w404 -> [w407 w417]
                    tunnel: [w408 w416] -> w402
                    frame 0, Default {
                      w411 = 1 items=["FreeRunning", "LockNext", "LockLatest"] ("mode")
                      # "Setup Camera Index"
                      # "Set grab mode"
                      # "Make Sure the camera is not running"
                      n521 = property class="IActiveFlyCapControl"(reference=w409, "Camera"=w410) -> (reference out=w412:refnum<k7>)  [unwired: 1 in, 1 out]
                      n522 = invoke class="IActiveFlyCapControl" method="ShowCamSlnModal"(reference=w412) -> (reference out=w414:refnum<k7>)  [unwired: 2 in, 2 out]
                      n523 = property class="IActiveFlyCapControl"(reference=w414, "Start"=0 ("Camera")) -> (reference out=w415:refnum<k7>)  [unwired: 1 in, 1 out]
                      n524 = invoke class="IActiveFlyCapControl" method="SetGrabMode"(reference=w415, "mode"=w411) -> (reference out=w408:refnum<k7>)  [unwired: 2 in, 3 out]
                    }
                    frame 1 {
                      w420 = 1 items=["FreeRunning", "LockNext", "LockLatest"] ("mode")
                      # "Setup Camera Index"
                      # "Set grab mode"
                      # "Make Sure the camera is not running"
                      n525 = property class="IActiveFlyCapControl"(reference=w417, "Camera"=w418) -> (reference out=w421:refnum<k7>)  [unwired: 1 in, 1 out]
                      n526 = invoke class="IActiveFlyCapControl" method="ShowCamSlnModal"(reference=w421) -> (reference out=w423:refnum<k7>)  [unwired: 2 in, 2 out]
                      n527 = property class="IActiveFlyCapControl"(reference=w423, "Start"=0 ("Camera")) -> (reference out=w424:refnum<k7>)  [unwired: 1 in, 1 out]
                      n528 = invoke class="IActiveFlyCapControl" method="SetGrabMode"(reference=w424, "mode"=w420) -> (reference out=w419:refnum<k7>)  [unwired: 2 in, 3 out]
                    }
                  }
                }
                n529 = local write "Initialize"(FALSE ("Initialize")) -> ()
                n530 = property on="Aquire" class="Bool (strict)"("DisabledEnum"=T1."Enabled" ("禁用")) -> ()  [unwired: 2 in, 2 out]
              }
              frame "CLE" {
                n531 = case shown="True" w427 {
                  tunnel: w430 -> [w435 w443]
                  tunnel: [w431 w441] -> w429
                  tunnel: w426 -> [w433 w440]
                  tunnel: [w434 w439] -> w425
                  frame False {
                    n532 = for {
                      N: 5 -> [_]
                      tunnel: [w438] -> w431
                      tunnel: w435 -> [w437]
                      tunnel: [w436] -> w434
                      tunnel: w433 -> [w436]
                      n533 = invoke class="IActiveFlyCapControl" method="GrabImage"(reference=w437) -> (reference out=w438:refnum<k7>)  [unwired: 2 in, 2 out]
                    }
                  }
                  frame True {
                    n534 = for {
                      N: 5 -> [_]
                      tunnel: w443 -> [w447]
                      tunnel: [w446] -> w441
                      tunnel: w440 -> [w445]
                      tunnel: [w444] -> w439
                      n535 = invoke class="IActiveFlyCapControl" method="GrabImage"(reference=w447) -> (reference out=w446:refnum<k7>)  [unwired: 2 in, 2 out]
                      n536 = invoke class="IActiveFlyCapControl" method="GrabImage"(reference=w445) -> (reference out=w444:refnum<k7>)  [unwired: 2 in, 2 out]
                    }
                  }
                }
                n537 = local write "Reset Cam Buffer"(FALSE ("Reset process index")) -> ()
              }
            }
          }
        }
        n538 = Wait Until Next ms Multiple(millisecond multiple=u32 100) -> ()  [unwired: 1 out]
      }
    }
    frame #2 {
      n539 = Release Queue(queue=w1039) -> ()  [unwired: 2 in, 3 out]
      n540 = Release Queue(queue=w1041) -> ()  [unwired: 2 in, 3 out]
      n541 = Release Queue(queue=w1040) -> ()  [unwired: 2 in, 3 out]
    }
  }
